vi "Image.vi"() -> ()   [LabVIEW 2017]
uses:
  ZaberTSeriesVI/Public/Utility/Request.ctl
  <vilib>/DAQmx/write.llb/DAQmx Write (Digital Bool 1Line 1Point).vi
  <vilib>/DAQmx/write.llb/DAQmx Write (Analog DBL 1Chan 1Samp).vi
  <vilib>/DAQmx/create/channels.llb/DAQmx Create Channel (AO-Voltage-Basic).vi
  <vilib>/DAQmx/miscellaneous.llb/DAQmx Fill In Error Info.vi
  <vilib>/DAQmx/create/channels.llb/DAQmx Create Channel (DO-Digital Output).vi
  <vilib>/Utility/file.llb/Read Delimited Spreadsheet (DBL).vi
  <vilib>/Utility/file.llb/Write Delimited Spreadsheet (string).vi
  <vilib>/Analysis/Matrix/Numeric/Conversions/Matrix To Array - RM.vi
  ZaberTSeriesVI/ZaberTSeries.lvlib
  <vilib>/Analysis/NI_AALPro.lvlib
  <vilib>/Analysis/Matrix/NI_Matrix.lvlib
panel:
  in  "Maximum offset":dbl=0.5
  out "WriteMS":bool=TRUE
  in  "Select PORT for LCQ":tag
  out "error out MS":errorcluster
  out "DAQmx Task MS":refnum<k21>
  in  "Stop MS":bool
  in  "scan range y [1E-7m]":dbl=282879.0 min=20.0 max=282879.0 step=2.0
  in  "scan range x [1E-7m]":dbl=282879.0 min=20.0 max=282879.0 step=2.0
  in  "File Export Path":path
  out "z(x) corrected":i32
  out "x corrected":i32
  out "zs":i32
  out "ys":i32
  out "xs":i32
  in  "Starting point":bool
  in  "Justage":bool
  out "error out Laserdiode":errorcluster
  in  "Request 11":T1={"Device Number"=0, "Command"=0, "Data"=0, "Response Count"=1} {"Command" items=["Echo"=55, "Home"=1, "Move Absolute"=20, "Move Relative"=21, "Move at Constant Speed"=22, "Renumber"=2, "Restore Settings"=36, "Stop"=23]}
  out "error out Stage":errorcluster
  in  "Refresh Button":bool
  out "ready.":bool
  out "Offset z(y) per µm":dbl
  out "Offset z(x) per µm":dbl
  out "z 3":i32
  out "z 2":i32
  out "z 1":i32
  in  "z [1E-7m]":i32=26400 min=0 max=282879 step=2
  in  "return to startpoint":bool
  out "x 3":i32
  out "y 3":i32
  out "x 2":i32
  out "y 2":i32
  in  "?":bool
  in  "?":bool
  out "Offset y per µm":dbl
  out "Offset x per µm":dbl
  in  "Calc Offset":bool
  in  "calibration":bool
  in  "Lens":enum16{"5x", "10x", "20x", "40x"}(ring)
  out "Read?":bool
  in  "Calib Path":path
  in  "Read Calibration file?":bool
  in  "intercept":dbl
  in  "slope":dbl
  in  "Shutter time (ms)":dbl=1.0 min=1.0 max=100000.0 step=1.0
  in  "y = step height [1E-7m]":dbl=2.0 min=2.0 max=282879.0 step=2.0
  in  "step scanning or continous (scan speed)":bool
  in  "Scan speed in µm/s":dbl=2.0 min=0.0 max=1000.0 step=2.0
  in  "End measurement":bool
  in  "x = step width [1E-7m]":dbl=2.0 min=2.0 max=282879.0 step=2.0
  in  "Begin measurement":bool
  out "error out shutter":errorcluster
  in  "Open/Close Shutter":bool
  in  "Select Channel for Shutter":tag
  out "y 1":i32
  out "x 1":i32
  in  "Turn on / off":bool
  in  "Set Zero":bool
  in  "Stop Laser":bool
  in  "stop Shutter":bool
  in  "Laserpower [W]":dbl(slide)=1e-08 min=0.0 max=1.0 step=0.1 scale=0.0..0.6
  in  "Select Channel for Laserdiode":tag
  out "position reached":bool
  in  "x [1E-7m]":i32 min=0 max=282879 step=2
  in  "Move":bool
  in  "y [1E-7m]":i32 min=0 max=282879 step=2
  in  "Stop Button":bool
  in  "Initialize Stage":bool
  in  "Select COM Port for Stage":refnum<visa-resource-name>
  out "DAQmx Task Shutter":refnum<k21>
  out "DAQmx Task Name Diode":refnum<k21>
  # "Imaging"
  # "Port 1, Line 0 = PFI0/P1.0"
  # "Set shutter to Xgate and Shutter enabled. Set Laserdiode controller to 0 mA and on. Make sure the stages manual knobs are in zero position. For calibration, a tab delimiter is used.\nNo plausibility check is performed on the calibration file!"
  # "!!TAKE CARE OF 5x vs 40x!!"
  # "CAREFUL! Init. will also reset z axis!!"
  # "Step height is a function of the temperature drift by desorption. In 10s@1300mA, ~1mm diameter is desorbed.\nPlease note: With scan speed, the outer limits are not perfectly timed. This is a numeric and electric issue and cannot be resolved"
  # "need to match\nmeas time in .seq\nfile"
  # "Please note it's 1E-7, not 1E-6!!"
  # "Before beginning the measurement, make sure you have set a shutter time, step height and width. Set your starting point and the calibration manually using this program and a camera. Save the position as it will be used for reset within the measurement!!!! \nCalibration: Set the offset positions properly. Take in mind that the stage moves towards positive values, therefore (0,0,0) must be lower than (0,y,0) and so on.\nClose the shutter, turn off Justage, then Turn on laser with the desired laser power, then hit begin measurement. If in measurement, the laser or shutter can be turned off using \"turn on/off\" button and the measurement can be stopped per axis using \"STOP\"."
  # "Offset listing"
  # "!!!! Set the calibration file for the laser power in backend: It is valid only for a specific optical path. Calibrate the laser power to the current in the experiment (have been measured for LD setup with microscope optics), then calculate intercept and slope and enter it as \"b\" and \"m\" according to y = mx+b in backend"
  # "0.5W = c.a. 900mA"
  # "This VI corrects the offset of the setup and substrate (e.g. rotation in the coating, tilt of slides,..) and the stage itself (1.2% moving too less per axis). The error in laser focus is additive in both x and y tilts and corrected as well. The stage error in z axis is only minor and cannot be corrected (1.2% of 100µm are 1.2µm < stage resolution - and this is already quite a lot)"
  # "x-, and y-value should be visible here, stating the current position (indicated by green light). \"Set zero\" sets the stage to absolute zero, but does not stop the measurement! \"Return to corrected zero\" returns the stage to bufff (x,y,z) = (0,0,0) starting point.  \"Calc offset\" corrects the xy- and xz-divergence on the spots and laser beam divergence on the substrate according to manually set calibration points.\n \nIf the measurements has finished, \"Begin measurement\" will go off and the stage will reset to buffered (x;y) or zero.\n\nSometimes the read current position will return the storing command. I don't know why. Workaround: Hit the button once more\n\nPlease note that if you pick scan speed, no export file will be written. From your starting point, the laser continously scans the substrate using the user-defined scan speed. The maximum travel distance of the stage is 28.2879 mm, minus the starting point, if defined. If required, remember that s=v*t.\n\nIf no export path is specified, the default path will be C:\\Users\\Username\\Documents\\LabVIEW Data\\"
  # "correct z with new justage"
  # "Bugtracker"
  # "Check laser spot correction in z with camera\n\nRead out current position sometimes returns\nreadout command\n."
  # "\"Maximum offset\" is the value that should not be exceed in the offset listing by any entry.\nAdjust only if necessary!"
  # "Zero corrected:"
  # "Disclaimer\nThis VI has not been excessively\ntested for safe use. Please use\nwith great care. \nalpha version without optimization"
  # "xz alignment:"
  # "yz alignment:"
  # "Error code stage:\n1 \tCannot Home \tHome - Device has traveled a long distance without triggering the home sensor. Device may be stalling or slipping.\n2 \tDevice Number Invalid \tRenumbering data out of range.\n14 \tVoltage Low \tPower supply voltage too low.\n15 \tVoltage High \tPower supply voltage too high.\n18 \tStored Position Invalid \tThe position stored in the requested register is no longer valid. This is probably because the maximum range was reduced.\n20 \tAbsolute Position Invalid \tMove Absolute - Target position out of range.\n21 \tRelative Position Invalid \tMove Relative - Target position out of range.\n22 \tVelocity Invalid \tConstant velocity move. Velocity out of range.\n36 \tPeripheral Id Invalid \tRestore Settings - peripheral id is invalid. Please use one of the peripheral ids listed in the user manual, or 0 for default.\n37 \tResolution Invalid \tInvalid microstep resolution. Resolution may only be 1, 2, 4, 8, 16, 32, 64, 128.\n38 \tRun Current Invalid \tRun current out of range. See command 38 for allowable values.\n39 \tHold Current Invalid \tHold current out of range. See command 39 for allowable values.\n40 \tMode Invalid \tSet Device Mode - one or more of the mode bits is invalid.\n41 \tHome Speed Invalid \tHome speed out of range. The range of home speed is determined by the resolution.\n42 \tSpeed Invalid \tTarget speed out of range. The range of target speed is determined by the resolution.\n43 \tAcceleration Invalid \tTarget acceleration out of range. The range of target acceleration is determined by the resolution.\n44 \tMaximum Range Invalid \tThe maximum range may only be set between 1 and the resolution limit of the stepper controller, which is 16,777,215.\n45 \tCurrent Position Invalid \tCurrent position out of range. Current position must be between 0 and the maximum range.\n46 \tMaximum Relative Move Invalid \tMax relative move out of range. Must be between 0 and 16,777,215.\n47 \tOffset Invalid \tHome offset out of range. Home offset must be between 0 and maximum range.\n48 \tAlias Invalid \tAlias out of range.\n49 \tLock State Invalid \tLock state must be 1 (locked) or 0 (unlocked).\n53 \tSetting Invalid \tReturn Setting - data entered is not a valid setting command number. Valid setting command numbers are the command numbers of any \"Set ...\" instructions.\n64 \tCommand Invalid \tCommand number not valid in this firmware version.\n255 \tBusy \tAnother command is executing and cannot be pre-empted. Either stop the previous command or wait until it finishes before trying again.\n1600 \tSave Position Invalid \tSave Current Position register out of range (must be 0-15).\n1601 \tSave Position Not Homed \tSave Current Position is not allowed unless the device has been homed.\n1700 \tReturn Position Invalid \tReturn Stored Position register out of range (must be 0-15).\n1800 \tMove Position Invalid \tMove to Stored Position register out of range (must be 0-15).\n1801 \tMove Position Not Homed \tMove to Stored Position is not allowed unless the device has been homed.\n2146 \tRelative Position Limited \tMove Relative (command 20) exceeded maximum relative move range. Either move a shorter distance, or change the maximum relative move (command 46).\n3600 \tSettings Locked \tMust clear Lock State (command 49) first. See the Set Lock State command for details.\n4008 \tDisable Auto Home Invalid \tSet Device Mode - this is a linear actuator; Disable Auto Home is used for rotary actuators only.\n4010 \tBit 10 Invalid \tSet Device Mode - bit 10 is reserved and must be 0.\n4012 \tHome Switch Invalid \tSet Device Mode - this device has integrated home sensor with preset polarity; mode bit 12 cannot be changed by the user.\n4013 \tBit 13 Invalid \tSet Device Mode - bit 13 is reserved and must be 0."
  # "Copyright (c) 2020 Alexander Knodel\n\nPermission is hereby granted, free of charge, to any person obtaining a copy\nof this software and associated documentation files (the \"Software\"), to deal\nin the Software without restriction, including without limitation the rights\nto use, copy, modify, merge, publish, distribute, sublicense, and/or sell\ncopies of the Software, and to permit persons to whom the Software is\nfurnished to do so, subject to the following conditions:\n\nThe above copyright notice and this permission notice shall be included in all\ncopies or substantial portions of the Software.\n\nTHE SOFTWARE IS PROVIDED \"AS IS\", WITHOUT WARRANTY OF ANY KIND, EXPRESS OR\nIMPLIED, INCLUDING BUT NOT LIMITED TO THE WARRANTIES OF MERCHANTABILITY,\nFITNESS FOR A PARTICULAR PURPOSE AND NONINFRINGEMENT. IN NO EVENT SHALL THE\nAUTHORS OR COPYRIGHT HOLDERS BE LIABLE FOR ANY CLAIM, DAMAGES OR OTHER\nLIABILITY, WHETHER IN AN ACTION OF CONTRACT, TORT OR OTHERWISE, ARISING FROM,\nOUT OF OR IN CONNECTION WITH THE SOFTWARE OR THE USE OR OTHER DEALINGS IN THE\nSOFTWARE."
types:
  T1 = typedef "ZaberTSeries.lvlib/Request.ctl" = cluster{"Device Number":u8, "Command":u8, "Data":i32, "Response Count":i32}
  T2 = typedef "ZaberTSeries.lvlib/Response.ctl" = cluster{"Device Number":u8, "Command":u8, "Data":i32}
  T3 = typedef "NI_Matrix.lvlib/RealMatrix.ctl" = dbl[][]
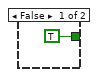
[diagram p2: hidden frame]
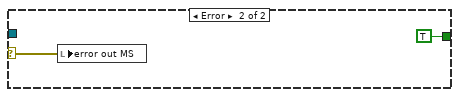
[diagram p3: hidden frame]
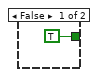
[diagram p4: hidden frame]
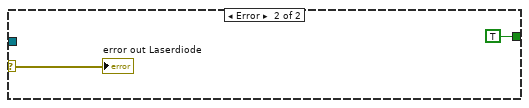
[diagram p5: hidden frame]
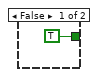
[diagram p6: hidden frame]
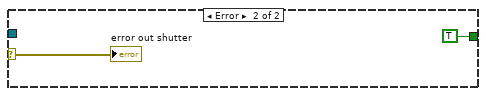
[diagram p7: hidden frame]
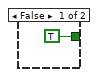
[diagram p8: hidden frame]
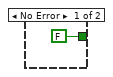
[diagram p9: hidden frame]
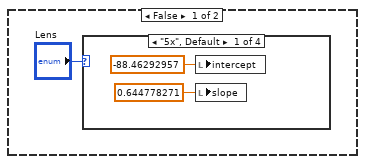
[diagram p10: hidden frame]
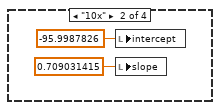
[diagram p11: hidden frame]
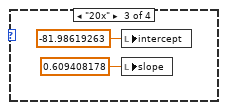
[diagram p12: hidden frame]
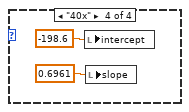
[diagram p13: hidden frame]
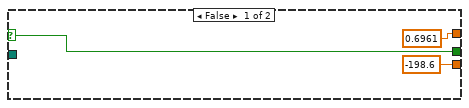
[diagram p14: hidden frame]
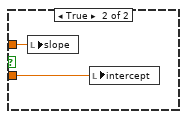
[diagram p15: hidden frame]
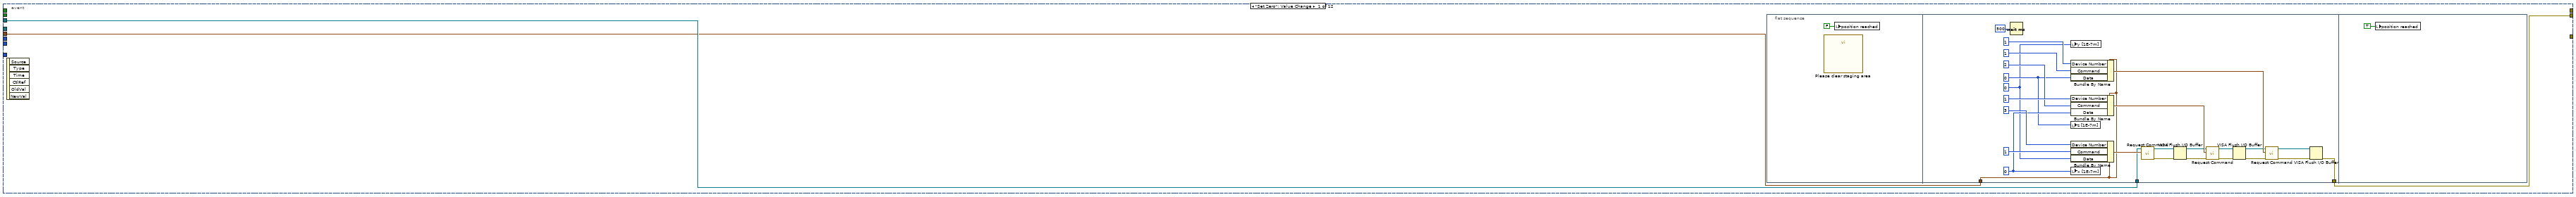
[diagram p16: hidden frame]
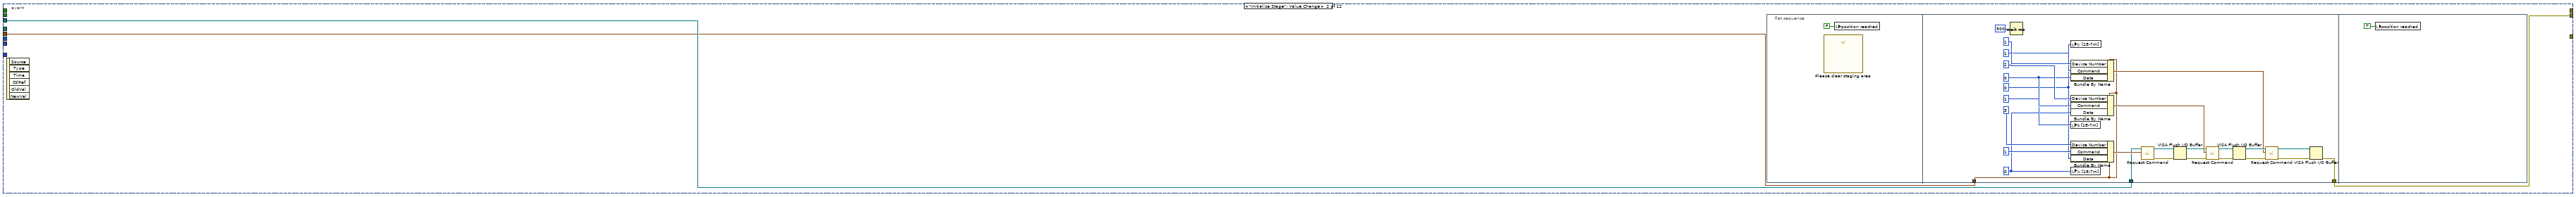
[diagram p17: hidden frame]
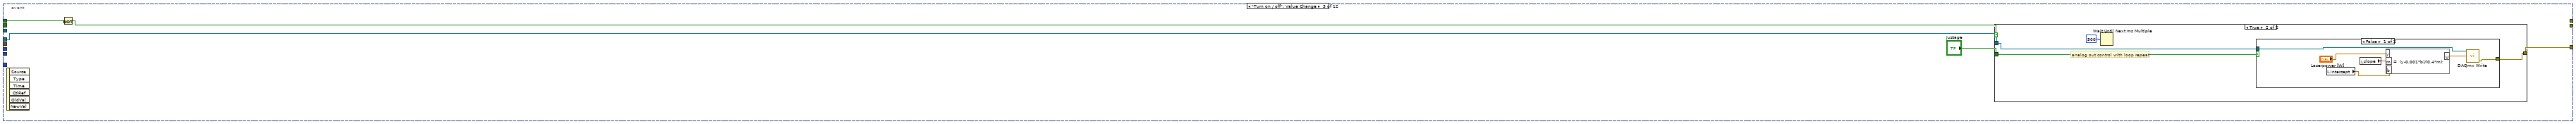
[diagram p18: hidden frame]
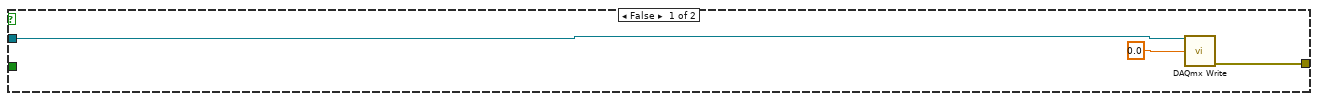
[diagram p19: hidden frame]
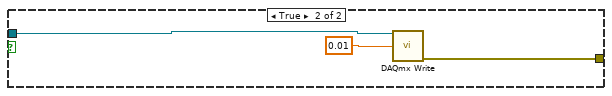
[diagram p20: hidden frame]
diagram:
  n1 = flat-sequence {
    tunnel: [w4] -> w2
    tunnel: w2 -> [w86]
    tunnel: [w86] -> w1
    tunnel: w1 -> [_]
    frame #0 {
      n2 = control-ref of="This VI"() -> (w3:refnum<vi>)
      n3 = invoke class="VI" method="Default Vals.Reinit All"(reference=w3) -> ()  [unwired: 2 in, 3 out]
    }
    frame #1 {
      n4 = while {
        stop <- w8 continue-if-true
        n5 = local read "Initialize Stage"() -> (w5:bool)
        n6 = Wait Until Next ms Multiple(millisecond multiple=u32 500) -> ()  [unwired: 1 out]
        n7 = case shown="True" w5 {
          tunnel: [TRUE w14] -> w7
          tunnel: "Select PORT for LCQ" -> [_ w13]
          frame False {
          }
          frame True {
            n8 = call-poly <vilib>:"DAQmx Create Virtual Channel.vi"("lines"=w13) -> ("task out"=w17:refnum<k21>, "error out"=w18:errorcluster)  [unwired: 13 in]
            n9 = call <vilib>:"DAQmx Start Task.vi"("task/channels in"=w17, "error in"=w18) -> ("task out"=w15:refnum<k21>, "error out"=w16:errorcluster)  [unwired: 12 in]
            "DAQmx Task MS" <- w15
            n10 = case shown="No Error" w16 {
              selector: w16 -> [_ w25]
              tunnel: w15 -> [w22 _]
              tunnel: [FALSE TRUE] -> w14
              frame No Error {
                n11 = call-poly <vilib>:"DAQmx Write.vi"("task/channels in"=w22, "data"=FALSE) -> ("error out"=→"error out MS":errorcluster)  [unwired: 11 in, 2 out]
                "WriteMS" <- TRUE
              }
              frame Error {
                n12 = local write "error out MS"(w25) -> ()
              }
            }
          }
        }
        n13 = Not(x="Stop MS") -> (.not. x?=w9:bool)
        n14 = And(x=w7, y=w9) -> (x .and. y?=w8:bool)
      }
      n15 = while {
        stop <- w27 continue-if-true
        # "initializes Slide Control to 0"
        n16 = Wait Until Next ms Multiple(millisecond multiple=u32 500) -> ()  [unwired: 1 out]
        n17 = local read "Initialize Stage"() -> (w26:bool)
        n18 = case shown="True" w26 {
          tunnel: "Select Channel for Laserdiode" -> [_ w37]
          tunnel: [TRUE w35] -> w31
          frame False {
          }
          frame True {
            n19 = call-poly <vilib>:"DAQmx Create Virtual Channel.vi"("physical channels"=w37) -> ("task out"=w39:refnum<k21>, "error out"=w38:errorcluster)  [unwired: 13 in]
            n20 = call <vilib>:"DAQmx Start Task.vi"("task/channels in"=w39, "error in"=w38) -> ("task out"=w34:refnum<k21>, "error out"=w36:errorcluster)  [unwired: 12 in]
            "DAQmx Task Name Diode" <- w34
            n21 = case shown="No Error" w36 {
              selector: w36 -> [_ w44]
              tunnel: [FALSE TRUE] -> w35
              tunnel: w34 -> [w41 _]
              frame No Error {
                n22 = call-poly <vilib>:"DAQmx Write.vi"("task/channels in"=w41, "data"=0.0) -> ("error out"=w42:errorcluster)  [unwired: 11 in, 2 out]
                n23 = local write "error out Laserdiode"(w42) -> ()
              }
              frame Error {
                "error out Laserdiode" <- w44
              }
            }
          }
        }
        n24 = Not(x="Stop Laser") -> (.not. x?=w30:bool)
        n25 = And(x=w31, y=w30) -> (x .and. y?=w27:bool)
      }
      n26 = while {
        stop <- w50 continue-if-true
        # "initializes Slide Control to 0"
        n27 = Wait Until Next ms Multiple(millisecond multiple=u32 500) -> ()  [unwired: 1 out]
        n28 = local read "Initialize Stage"() -> (w46:bool)
        n29 = case shown="True" w46 {
          tunnel: "Select Channel for Shutter" -> [_ w56]
          tunnel: [TRUE w61] -> w49
          frame False {
          }
          frame True {
            # "Make sure Shutter in on, on X Gate and enabled"
            n30 = call-poly <vilib>:"DAQmx Create Virtual Channel.vi"("maximum value"=5.0, "minimum value"=0.0, "physical channels"=w56) -> ("task out"=w58:refnum<k21>, "error out"=w57:errorcluster)  [unwired: 11 in]
            n31 = call <vilib>:"DAQmx Start Task.vi"("task/channels in"=w58, "error in"=w57) -> ("task out"=w54:refnum<k21>, "error out"=w55:errorcluster)  [unwired: 12 in]
            "DAQmx Task Shutter" <- w54
            n32 = case shown="No Error" w55 {
              selector: w55 -> [_ w66]
              tunnel: [FALSE TRUE] -> w61
              tunnel: w54 -> [w64 _]
              frame No Error {
                n33 = call-poly <vilib>:"DAQmx Write.vi"("task/channels in"=w64, "data"=0.0) -> ("error out"=w63:errorcluster)  [unwired: 11 in, 2 out]
                n34 = local write "error out shutter"(w63) -> ()
              }
              frame Error {
                "error out shutter" <- w66
              }
            }
          }
        }
        n35 = Not(x="stop Shutter") -> (.not. x?=w51:bool)
        n36 = And(x=w49, y=w51) -> (x .and. y?=w50:bool)
      }
      n37 = while {
        tunnel: ["Stop Button"] -> w4
        stop <- w70 continue-if-true
        n38 = Wait Until Next ms Multiple(millisecond multiple=u32 500) -> ()  [unwired: 1 out]
        n39 = case shown="True" "Initialize Stage" {
          tunnel: [TRUE w82] -> w72
          tunnel: "Select COM Port for Stage" -> [_ w79]
          frame False {
          }
          frame True {
            n40 = call "Initialize.vi"("VISA resource name"=w79) -> ("error out"=w81:errorcluster, "VISA resource name out"=w76:refnum<visa-resource-name>)  [unwired: 8 in, 1 out]
            n41 = property class="Instr"(reference=w76, error in=w81, "Timeout"=u32 30000 ("General Settings:Timeout Value")) -> (reference out=w77:refnum<visa-resource-name>, error out=w78:errorcluster)
            n42 = local write "Select COM Port for Stage"(w77) -> ()
            n43 = case shown="Error" w78 {
              selector: w78 -> [_ w84]
              tunnel: [FALSE TRUE] -> w82
              frame No Error {
              }
              frame Error {
                "error out Stage" <- w84
              }
            }
          }
        }
        n44 = Not(x="Stop Button") -> (.not. x?=w71:bool)
        n45 = And(x=w72, y=w71) -> (x .and. y?=w70:bool)
      }
    }
    frame #2 {
      n46 = flat-sequence {
        frame #0 {
          n47 = case shown="True" "Read Calibration file?" {
            tunnel: "Calib Path" -> [_ w98]
            frame False {
              n48 = case shown="\"5x\", Default" "Lens" {
                frame "5x", Default {
                  n49 = local write "intercept"(-88.46292957 ("input variable")) -> ()
                  n50 = local write "slope"(0.644778271 ("input variable")) -> ()
                }
                frame "10x" {
                  n51 = local write "intercept"(-95.9987826 ("input variable")) -> ()
                  n52 = local write "slope"(0.709031415 ("input variable")) -> ()
                }
                frame "20x" {
                  n53 = local write "intercept"(-81.98619263 ("input variable")) -> ()
                  n54 = local write "slope"(0.609408178 ("input variable")) -> ()
                }
                frame "40x" {
                  n55 = local write "intercept"(-198.6 ("intercept")) -> ()
                  n56 = local write "slope"(0.6961 ("slope")) -> ()
                }
              }
            }
            frame True {
              n57 = flat-sequence {
                tunnel: [w103] -> w99
                tunnel: w98 -> [w103]
                tunnel: [w104] -> w102
                tunnel: [w108] -> w101
                tunnel: [w107] -> w100
                tunnel: w99 -> [w105]
                tunnel: w102 -> [w127]
                tunnel: w101 -> [w126]
                tunnel: w100 -> [w125]
                frame #0 {
                }
                frame #1 {
                  n58 = call <vilib>:"Is Path and Not Empty.vi"("path"=w105) -> ("Is Path and Not Empty?"=w109:bool)  [unwired: 4 in]
                  n59 = Wait (ms)(milliseconds to wait=u32 500) -> ()  [unwired: 1 out]
                  n60 = case shown="True" w109 {
                    selector: w109 -> [w110 _]
                    tunnel: w105 -> [_ w117]
                    tunnel: [0.6961 ("slope") w115] -> w107
                    tunnel: [-198.6 ("intercept") w116] -> w108
                    tunnel: [w110 w113] -> w104
                    frame False {
                    }
                    frame True {
                      n61 = call-poly <vilib>:"Read Delimited Spreadsheet.vi"("file path (dialog if empty)"=w117) -> ("all rows"=w120:dbl[][], "EOF?"=→"Read?":bool, "error out"=w118:errorcluster)  [unwired: 9 in, 3 out]
                      n62 = local write "error out Laserdiode"(w118) -> ()
                      n63 = Index Array(array=w120, index (col)=1 ("disabled index (col)")) -> (element=w124:dbl[])  [unwired: 1 in]
                      n64 = Index Array(array=w120, index (col)=0 ("disabled index (col)")) -> (element=w123:dbl[])  [unwired: 1 in]
                      n65 = call <vilib>:"Linear Fit.vi"("Y"=w124, "X"=w123) -> ("slope"=w115:dbl, "intercept"=w116:dbl)  [unwired: 9 in, 3 out]
                      n66 = Not A Number/Path/Refnum?(number/path/refnum=w116) -> (NaN/Path/Refnum?=w114:bool)
                      n67 = Not(x=w114) -> (.not. x?=w113:bool)
                    }
                  }
                }
                frame #2 {
                  n68 = case shown="False" w127 {
                    tunnel: w126 -> [_ w130]
                    tunnel: w125 -> [_ w131]
                    frame False {
                      n69 = call "Display Message to User"() -> ()  [unwired: 10 in, 2 out]
                      n70 = local write "intercept"(-198.6 ("intercept")) -> ()
                      n71 = local write "slope"(0.6961 ("slope")) -> ()
                    }
                    frame True {
                      n72 = local write "slope"(w131) -> ()
                      n73 = local write "intercept"(w130) -> ()
                    }
                  }
                }
              }
            }
          }
        }
      }
    }
    frame #3 {
      n74 = flat-sequence {
        tunnel: [w137] -> w133
        tunnel: [w134] -> w132
        tunnel: w133 -> [w1147]
        tunnel: w132 -> [w1146]
        frame #0 {
          n75 = local read "Select COM Port for Stage"() -> (w135:refnum<visa-resource-name>)
          n76 = while {
            tunnel: "Request 11" -> [w146]
            tunnel: w135 -> [w145]
            stop <- w147 stop-if-true
            n77 = local read "position reached"() -> (→"ready.":bool)
            n78 = local read "DAQmx Task Name Diode"() -> (w139:refnum<k21>)
            n79 = Wait Until Next ms Multiple(millisecond multiple=u32 500) -> ()  [unwired: 1 out]
            n80 = Not(x="Open/Close Shutter") -> (.not. x?=w142:bool)
            n81 = event shown="[9] \"Refresh Button\": Value Change" {
              selector: _ -> [_ _ _ _ _ _ _ _ _ _ _ _]
              dyn-events: _ -> [_ _ _ _ _ _ _ _ _ _ _ _]
              timeout: _ -> [_ _ _ _ _ _ _ _ _ _ _ _]
              tunnel: [w154 w185 _ w237 _ _ _ _ w322 w353 _ w447] -> w144
              tunnel: w145 -> [w155 w186 _ w238 _ _ _ _ w321 w352 _ w448]
              tunnel: "x [1E-7m]" -> [_ _ _ _ w307 w309 w312 w315 w320 _ _ _]
              tunnel: "y [1E-7m]" -> [_ _ _ _ w306 w310 w313 w316 w319 _ _ _]
              tunnel: "z [1E-7m]" -> [_ _ _ _ w305 w308 w311 w314 w318 _ _ _]
              tunnel: w142 -> [_ _ _ _ _ _ _ _ _ _ w443 _]
              tunnel: w146 -> [w153 w184 _ w236 _ _ _ _ w317 w351 _ w446]
              tunnel: [_ _ _ _ _ _ _ _ _ _ w440 _] -> w141
              tunnel: "Turn on / off" -> [_ _ w217 _ _ _ _ _ _ _ _ _]
              tunnel: [_ _ w219 _ _ _ _ _ _ _ _ _] -> w140
              tunnel: w139 -> [_ _ w218 _ _ _ _ _ _ _ _ _]
              event "Set Zero": Value Change {
                n82 = event-data() -> ()  [unwired: 1 in, 6 out]
                n83 = flat-sequence {
                  tunnel: w155 -> [w166]
                  tunnel: [w163] -> w154
                  tunnel: w153 -> [w160]
                  frame #0 {
                    n84 = call "Please clear staging area"() -> ()  [unwired: 18 in, 2 out]
                    n85 = local write "position reached"(FALSE ("Blinking")) -> ()
                  }
                  frame #1 {
                    w158 = 0 ("y-value 2")
                    w159 = 0 ("y-value 2")
                    w157 = 0 ("x-value 2")
                    n86 = Wait (ms)(milliseconds to wait=u32 500 ("millisecond timer value")) -> ()  [unwired: 1 out]
                    n87 = local write "y [1E-7m]"(w157) -> ()
                    n88 = Bundle By Name(cluster=w160, "Device Number"=u8 1, "Command"=u8 1, "Data"=w158) -> (w168:T1)
                    n89 = Bundle By Name(cluster=w160, "Device Number"=u8 2, "Command"=u8 1, "Data"=w159) -> (w177:T1)
                    n90 = local write "z [1E-7m]"(w158) -> ()
                    n91 = Bundle By Name(cluster=w160, "Device Number"=u8 3, "Command"=u8 1, "Data"=w157) -> (w180:T1)
                    n92 = local write "x [1E-7m]"(w159) -> ()
                    n93 = call "Request Command.vi"("Request"=w180, "VISA resource name"=w166) -> ("error out"=w182:errorcluster, "VISA resource name out"=w181:refnum<visa-resource-name>)  [unwired: 6 in, 2 out]
                    n94 = VISA Flush I/O Buffer(VISA resource name=w181, error in (no error)=w182) -> (VISA resource name out=w176:refnum<visa-resource-name>, error out=w175:errorcluster)  [unwired: 1 in]
                    n95 = call "Request Command.vi"("error in (no error)"=w175, "Request"=w177, "VISA resource name"=w176) -> ("error out"=w171:errorcluster, "VISA resource name out"=w172:refnum<visa-resource-name>)  [unwired: 5 in, 2 out]
                    n96 = VISA Flush I/O Buffer(VISA resource name=w172, error in (no error)=w171) -> (VISA resource name out=w164:refnum<visa-resource-name>, error out=w162:errorcluster)  [unwired: 1 in]
                    n97 = call "Request Command.vi"("error in (no error)"=w162, "Request"=w168, "VISA resource name"=w164) -> ("error out"=w165:errorcluster, "VISA resource name out"=w167:refnum<visa-resource-name>)  [unwired: 5 in, 2 out]
                    n98 = VISA Flush I/O Buffer(VISA resource name=w167, error in (no error)=w165) -> (error out=w163:errorcluster)  [unwired: 1 in, 1 out]
                  }
                  frame #2 {
                    n99 = local write "position reached"(TRUE ("Blinking")) -> ()
                  }
                }
              }
              event "Initialize Stage": Value Change {
                n100 = event-data() -> ()  [unwired: 1 in, 6 out]
                n101 = flat-sequence {
                  tunnel: w186 -> [w201]
                  tunnel: [w198] -> w185
                  tunnel: w184 -> [w191]
                  frame #0 {
                    n102 = call "Please clear staging area"() -> ()  [unwired: 18 in, 2 out]
                    n103 = local write "position reached"(FALSE ("Blinking")) -> ()
                  }
                  frame #1 {
                    w190 = 0 ("Data")
                    w189 = 0 ("y-value 2")
                    w188 = 0 ("x-value 2")
                    n104 = Wait (ms)(milliseconds to wait=u32 500 ("millisecond timer value")) -> ()  [unwired: 1 out]
                    n105 = local write "y [1E-7m]"(w188) -> ()
                    n106 = Bundle By Name(cluster=w191, "Device Number"=u8 1, "Command"=u8 1, "Data"=w190) -> (w193:T1)
                    n107 = Bundle By Name(cluster=w191, "Device Number"=u8 2, "Command"=u8 1, "Data"=w189) -> (w208:T1)
                    n108 = local write "z [1E-7m]"(w190) -> ()
                    n109 = Bundle By Name(cluster=w191, "Device Number"=u8 3, "Command"=u8 1, "Data"=w188) -> (w211:T1)
                    n110 = local write "x [1E-7m]"(w189) -> ()
                    n111 = call "Request Command.vi"("Request"=w211, "VISA resource name"=w201) -> ("error out"=w213:errorcluster, "VISA resource name out"=w212:refnum<visa-resource-name>)  [unwired: 6 in, 2 out]
                    n112 = VISA Flush I/O Buffer(VISA resource name=w212, error in (no error)=w213) -> (VISA resource name out=w207:refnum<visa-resource-name>, error out=w206:errorcluster)  [unwired: 1 in]
                    n113 = call "Request Command.vi"("error in (no error)"=w206, "Request"=w208, "VISA resource name"=w207) -> ("error out"=w202:errorcluster, "VISA resource name out"=w203:refnum<visa-resource-name>)  [unwired: 5 in, 2 out]
                    n114 = VISA Flush I/O Buffer(VISA resource name=w203, error in (no error)=w202) -> (VISA resource name out=w194:refnum<visa-resource-name>, error out=w195:errorcluster)  [unwired: 1 in]
                    n115 = call "Request Command.vi"("error in (no error)"=w195, "Request"=w193, "VISA resource name"=w194) -> ("error out"=w196:errorcluster, "VISA resource name out"=w197:refnum<visa-resource-name>)  [unwired: 5 in, 2 out]
                    n116 = VISA Flush I/O Buffer(VISA resource name=w197, error in (no error)=w196) -> (error out=w198:errorcluster)  [unwired: 1 in, 1 out]
                  }
                  frame #2 {
                    n117 = local write "position reached"(TRUE ("Blinking")) -> ()
                  }
                }
              }
              event "Turn on / off": Value Change {
                n118 = event-data() -> ()  [unwired: 1 in, 6 out]
                n119 = Not(x=w217) -> (.not. x?=w216:bool)
                n120 = case shown="True" w216 {
                  tunnel: w218 -> [w222 w225]
                  tunnel: [w220 w224] -> w219
                  tunnel: "Justage" -> [_ w223]
                  frame False {
                    n121 = call-poly <vilib>:"DAQmx Write.vi"("task/channels in"=w222, "data"=0.0) -> ("error out"=w220:errorcluster)  [unwired: 11 in, 2 out]
                  }
                  frame True {
                    # "analog out control with loop repeat"
                    n122 = Wait Until Next ms Multiple(millisecond multiple=u32 500) -> ()  [unwired: 1 out]
                    n123 = case shown="False" w223 {
                      tunnel: [w229 w234] -> w224
                      tunnel: w225 -> [w227 w235]
                      frame False {
                        n124 = local read "intercept"() -> (w230:dbl)
                        n125 = local read "slope"() -> (w231:dbl)
                        n126 = formula code="U =  (y-0.001*b)/(0.4*m);"("y"="Laserpower [W]", "m"=w231, "b"=w230) -> ("U"=w228:dbl)
                        n127 = call-poly <vilib>:"DAQmx Write.vi"("task/channels in"=w227, "data"=w228) -> ("error out"=w229:errorcluster)  [unwired: 11 in, 2 out]
                      }
                      frame True {
                        n128 = call-poly <vilib>:"DAQmx Write.vi"("task/channels in"=w235, "data"=0.01) -> ("error out"=w234:errorcluster)  [unwired: 11 in, 2 out]
                      }
                    }
                  }
                }
              }
              event "return to startpoint": Value Change {
                n129 = event-data() -> ()  [unwired: 1 in, 6 out]
                n130 = flat-sequence {
                  tunnel: w238 -> [w257]
                  tunnel: [w254] -> w237
                  tunnel: w236 -> [w251]
                  frame #0 {
                    n131 = local write "position reached"(FALSE ("Blinking")) -> ()
                  }
                  frame #1 {
                    n132 = local read "zs"() -> (w244:i32)
                    n133 = local read "xs"() -> (w245:i32)
                    n134 = local read "ys"() -> (w243:i32)
                    n135 = Wait (ms)(milliseconds to wait=u32 500 ("millisecond timer value")) -> ()  [unwired: 1 out]
                    n136 = Not Equal To 0?(x=w244) -> (x != 0?=w248:bool)
                    n137 = Not Equal To 0?(x=w245) -> (x != 0?=w250:bool)
                    n138 = Not Equal To 0?(x=w243) -> (x != 0?=w249:bool)
                    n139 = Build Array(w250, w249, w248) -> (w247:bool[])
                    n140 = And Array Elements(Boolean array=w247) -> (logical AND=w246:bool)
                    n141 = case shown="True" w246 {
                      tunnel: [w275 w301] -> w241
                      tunnel: [w274 w302] -> w240
                      tunnel: [w278 w303] -> w242
                      tunnel: w245 -> [_ w303]
                      tunnel: w243 -> [_ w302]
                      tunnel: w244 -> [_ w301]
                      frame False {
                        n142 = local read "z 1"() -> (w276:i32)
                        n143 = local read "x 1"() -> (w279:i32)
                        n144 = local read "y 1"() -> (w277:i32)
                        n145 = Build Array(w279, w277, w276) -> (w282:i32[])
                        n146 = Not Equal To 0?(x=w282) -> (x != 0?=w281:bool[])
                        n147 = And Array Elements(Boolean array=w281) -> (logical AND=w280:bool)
                        n148 = case shown="True" w280 {
                          tunnel: [w288 w300] -> w278
                          tunnel: w279 -> [_ w300]
                          tunnel: w277 -> [_ w299]
                          tunnel: [w286 w299] -> w274
                          tunnel: w276 -> [_ w298]
                          tunnel: [w284 w298] -> w275
                          frame False {
                            n149 = local read "error out Stage"() -> (w291:errorcluster)
                            n150 = call "Warning! You may ruin your measurement (no start. point)"("error in (no error)"=w291) -> ("z"=w285:dbl, "y"=w287:dbl, "x"=w289:dbl, "OK"=w283:bool, "error out"=w290:errorcluster)  [unwired: 14 in]
                            n151 = local write "error out Stage"(w290) -> ()
                            n152 = case shown="True" w283 {
                              tunnel: w289 -> [_ w295]
                              tunnel: [w292 w295] -> w288
                              tunnel: [w292 w294] -> w286
                              tunnel: w287 -> [_ w294]
                              tunnel: w285 -> [_ w293]
                              tunnel: [w292 w293] -> w284
                              frame False {
                                w292 = 0
                              }
                              frame True {
                              }
                            }
                          }
                          frame True {
                            n153 = local read "error out Stage"() -> (w297:errorcluster)
                            n154 = call "Display Message to User4"("error in (no error)"=w297) -> ("error out"=w296:errorcluster)  [unwired: 9 in, 1 out]
                            n155 = local write "error out Stage"(w296) -> ()
                          }
                        }
                      }
                      frame True {
                      }
                    }
                    n156 = local write "z [1E-7m]"(w241) -> ()
                    n157 = local write "x [1E-7m]"(w242) -> ()
                    n158 = local write "y [1E-7m]"(w240) -> ()
                    n159 = Bundle By Name(cluster=w251, "Device Number"=u8 1, "Command"=u8 20, "Data"=w241) -> (w259:T1)
                    n160 = Bundle By Name(cluster=w251, "Device Number"=u8 2, "Command"=u8 20, "Data"=w242) -> (w268:T1)
                    n161 = Bundle By Name(cluster=w251, "Device Number"=u8 3, "Command"=u8 20, "Data"=w240) -> (w271:T1)
                    n162 = call "Request Command.vi"("Request"=w271, "VISA resource name"=w257) -> ("error out"=w273:errorcluster, "VISA resource name out"=w272:refnum<visa-resource-name>)  [unwired: 6 in, 2 out]
                    n163 = VISA Flush I/O Buffer(VISA resource name=w272, error in (no error)=w273) -> (VISA resource name out=w267:refnum<visa-resource-name>, error out=w266:errorcluster)  [unwired: 1 in]
                    n164 = call "Request Command.vi"("error in (no error)"=w266, "Request"=w268, "VISA resource name"=w267) -> ("error out"=w262:errorcluster, "VISA resource name out"=w263:refnum<visa-resource-name>)  [unwired: 5 in, 2 out]
                    n165 = VISA Flush I/O Buffer(VISA resource name=w263, error in (no error)=w262) -> (VISA resource name out=w255:refnum<visa-resource-name>, error out=w253:errorcluster)  [unwired: 1 in]
                    n166 = call "Request Command.vi"("error in (no error)"=w253, "Request"=w259, "VISA resource name"=w255) -> ("error out"=w256:errorcluster, "VISA resource name out"=w258:refnum<visa-resource-name>)  [unwired: 5 in, 2 out]
                    n167 = VISA Flush I/O Buffer(VISA resource name=w258, error in (no error)=w256) -> (error out=w254:errorcluster)  [unwired: 1 in, 1 out]
                  }
                  frame #2 {
                    n168 = local write "position reached"(TRUE ("Blinking")) -> ()
                  }
                }
              }
              event "calibration": Value Change {
                n169 = event-data() -> ()  [unwired: 1 in, 6 out]
                "x 1" <- w307
                "y 1" <- w306
                "z 1" <- w305
              }
              event Value Change {
                n170 = event-data() -> ()  [unwired: 1 in, 6 out]
                "y 2" <- w310
                "x 2" <- w309
                "z 2" <- w308
              }
              event Value Change {
                n171 = event-data() -> ()  [unwired: 1 in, 6 out]
                "x 3" <- w312
                "y 3" <- w313
                "z 3" <- w311
              }
              event "Starting point": Value Change {
                n172 = event-data() -> ()  [unwired: 1 in, 6 out]
                "zs" <- w314
                "ys" <- w316
                "xs" <- w315
              }
              event "Move": Value Change {
                n173 = event-data() -> ()  [unwired: 1 in, 5 out]
                n174 = flat-sequence {
                  tunnel: [w336] -> w322
                  tunnel: w321 -> [w337]
                  tunnel: w320 -> [w324]
                  tunnel: w319 -> [w325]
                  tunnel: w318 -> [w326]
                  tunnel: w317 -> [w327]
                  frame #0 {
                    n175 = local write "position reached"(FALSE ("Blinking")) -> ()
                  }
                  frame #1 {
                    n176 = Wait (ms)(milliseconds to wait=u32 500 ("millisecond timer value")) -> ()  [unwired: 1 out]
                    n177 = Bundle By Name(cluster=w327, "Device Number"=u8 1, "Command"=u8 20, "Data"=w326) -> (w331:T1)
                    n178 = Bundle By Name(cluster=w327, "Device Number"=u8 2, "Command"=u8 20, "Data"=w324) -> (w344:T1)
                    n179 = Bundle By Name(cluster=w327, "Device Number"=u8 3, "Command"=u8 20, "Data"=w325) -> (w347:T1)
                    n180 = call "Request Command.vi"("Request"=w347, "VISA resource name"=w337) -> ("error out"=w349:errorcluster, "VISA resource name out"=w348:refnum<visa-resource-name>)  [unwired: 6 in, 2 out]
                    n181 = VISA Flush I/O Buffer(VISA resource name=w348, error in (no error)=w349) -> (VISA resource name out=w343:refnum<visa-resource-name>, error out=w342:errorcluster)  [unwired: 1 in]
                    n182 = call "Request Command.vi"("error in (no error)"=w342, "Request"=w344, "VISA resource name"=w343) -> ("error out"=w338:errorcluster, "VISA resource name out"=w339:refnum<visa-resource-name>)  [unwired: 5 in, 2 out]
                    n183 = VISA Flush I/O Buffer(VISA resource name=w339, error in (no error)=w338) -> (VISA resource name out=w333:refnum<visa-resource-name>, error out=w335:errorcluster)  [unwired: 1 in]
                    n184 = call "Request Command.vi"("error in (no error)"=w335, "Request"=w331, "VISA resource name"=w333) -> ("error out"=w334:errorcluster, "VISA resource name out"=w332:refnum<visa-resource-name>)  [unwired: 5 in, 2 out]
                    n185 = VISA Flush I/O Buffer(VISA resource name=w332, error in (no error)=w334) -> (error out=w336:errorcluster)  [unwired: 1 in, 1 out]
                  }
                  frame #2 {
                    n186 = local write "position reached"(TRUE ("Blinking")) -> ()
                  }
                }
              }
              event "Refresh Button": Value Change {
                n187 = event-data() -> ()  [unwired: 1 in, 6 out]
                n188 = while {
                  tunnel: [w360] -> w353
                  tunnel: w352 -> [w359]
                  tunnel: w351 -> [w358]
                  i -> [w356]
                  stop <- w354 continue-if-true
                  n189 = Equal?(x=w356, y=4.0) -> (x = y?=w355:bool)
                  n190 = flat-sequence {
                    tunnel: [w366] -> w360
                    tunnel: w355 -> [w362]
                    tunnel: w359 -> [w365]
                    tunnel: w358 -> [w364]
                    tunnel: [w361] -> w354
                    frame #0 {
                      n191 = flat-sequence {
                        tunnel: [w372] -> w368
                        tunnel: [w371] -> w367
                        tunnel: w365 -> [w370]
                        tunnel: w364 -> [w369]
                        tunnel: w368 -> [w398]
                        tunnel: w367 -> [w397]
                        tunnel: w364 -> [w396]
                        tunnel: [w399] -> w363
                        tunnel: [w438] -> w366
                        tunnel: w363 -> [w438]
                        tunnel: w362 -> [w437]
                        tunnel: [w430] -> w361
                        frame #0 {
                          n192 = Bundle By Name(cluster=w369, "Device Number"=u8 3, "Command"=u8 16, "Data"=2) -> (w393:T1)
                          n193 = Bundle By Name(cluster=w369, "Device Number"=u8 2, "Command"=u8 16, "Data"=1) -> (w387:T1)
                          n194 = Bundle By Name(cluster=w369, "Device Number"=u8 1, "Command"=u8 16, "Data"=0) -> (w383:T1)
                          n195 = Wait (ms)(milliseconds to wait=u32 2000 ("millisecond timer value")) -> ()  [unwired: 1 out]
                          n196 = call "Request Command.vi"("Request"=w383, "VISA resource name"=w370) -> ("error out"=w381:errorcluster, "VISA resource name out"=w382:refnum<visa-resource-name>)  [unwired: 6 in, 2 out]
                          n197 = VISA Flush I/O Buffer(VISA resource name=w382, error in (no error)=w381) -> (VISA resource name out=w376:refnum<visa-resource-name>, error out=w373:errorcluster)  [unwired: 1 in]
                          n198 = call "Request Command.vi"("error in (no error)"=w373, "Request"=w387, "VISA resource name"=w376) -> ("error out"=w388:errorcluster, "VISA resource name out"=w389:refnum<visa-resource-name>)  [unwired: 5 in, 2 out]
                          n199 = VISA Flush I/O Buffer(VISA resource name=w389, error in (no error)=w388) -> (VISA resource name out=w375:refnum<visa-resource-name>, error out=w374:errorcluster)  [unwired: 1 in]
                          n200 = call "Request Command.vi"("error in (no error)"=w374, "Request"=w393, "VISA resource name"=w375) -> ("error out"=w395:errorcluster, "VISA resource name out"=w394:refnum<visa-resource-name>)  [unwired: 5 in, 2 out]
                          n201 = VISA Flush I/O Buffer(VISA resource name=w394, error in (no error)=w395) -> (VISA resource name out=w371:refnum<visa-resource-name>, error out=w372:errorcluster)  [unwired: 1 in]
                        }
                        frame #1 {
                          n202 = Wait (ms)(milliseconds to wait=u32 2000 ("millisecond timer value")) -> ()  [unwired: 1 out]
                          n203 = Bundle By Name(cluster=w396, "Device Number"=u8 2, "Command"=u8 17, "Data"=1) -> (w409:T1)
                          n204 = Bundle By Name(cluster=w396, "Device Number"=u8 3, "Command"=u8 17, "Data"=2) -> (w424:T1)
                          n205 = Bundle By Name(cluster=w396, "Device Number"=u8 1, "Command"=u8 17, "Data"=0) -> (w423:T1)
                          n206 = call "Request Command.vi"("error in (no error)"=w398, "Request"=w423, "VISA resource name"=w397) -> ("error out"=w425:errorcluster, "First Response"=w412:T2, "VISA resource name out"=w428:refnum<visa-resource-name>)  [unwired: 5 in, 1 out]
                          n207 = Unbundle(w412) -> ("Data"=w410:i32)  [unwired: 2 out]
                          n208 = VISA Flush I/O Buffer(VISA resource name=w428, error in (no error)=w425) -> (VISA resource name out=w405:refnum<visa-resource-name>, error out=w404:errorcluster)  [unwired: 1 in]
                          n209 = local write "z [1E-7m]"(w410) -> ()
                          n210 = call "Request Command.vi"("error in (no error)"=w404, "Request"=w424, "VISA resource name"=w405) -> ("error out"=w426:errorcluster, "First Response"=w411:T2, "VISA resource name out"=w427:refnum<visa-resource-name>)  [unwired: 5 in, 1 out]
                          n211 = Unbundle(w411) -> ("Data"=w400:i32)  [unwired: 2 out]
                          n212 = VISA Flush I/O Buffer(VISA resource name=w427, error in (no error)=w426) -> (VISA resource name out=w402:refnum<visa-resource-name>, error out=w403:errorcluster)  [unwired: 1 in]
                          n213 = local write "y [1E-7m]"(w400) -> ()
                          n214 = call "Request Command.vi"("error in (no error)"=w403, "Request"=w409, "VISA resource name"=w402) -> ("error out"=w406:errorcluster, "First Response"=w407:T2, "VISA resource name out"=w408:refnum<visa-resource-name>)  [unwired: 5 in, 1 out]
                          n215 = Unbundle(w407) -> ("Data"=w401:i32)  [unwired: 2 out]
                          n216 = VISA Flush I/O Buffer(VISA resource name=w408, error in (no error)=w406) -> (error out=w399:errorcluster)  [unwired: 1 in, 1 out]
                          n217 = local write "x [1E-7m]"(w401) -> ()
                        }
                        frame #2 {
                          n218 = local read "z [1E-7m]"() -> (w436:i32)
                          n219 = local read "y [1E-7m]"() -> (w435:i32)
                          n220 = local read "x [1E-7m]"() -> (w434:i32)
                          n221 = Wait (ms)(milliseconds to wait=u32 500 ("millisecond timer value")) -> ()  [unwired: 1 out]
                          n222 = Build Array(w436, w435, w434) -> (w433:i32[])
                          n223 = Less Or Equal?(x=w433, y=2) -> (x <= y?=w432:bool[])
                          n224 = case shown="True" w437 {
                            frame False {
                            }
                            frame True {
                              n225 = call "Display Message to User3"() -> ("error out"=w439:errorcluster)  [unwired: 10 in, 1 out]
                              n226 = local write "error out Stage"(w439) -> ()
                            }
                          }
                          n227 = Or Array Elements(Boolean array=w432) -> (logical OR=w430:bool)
                        }
                      }
                    }
                  }
                }
              }
              event "Open/Close Shutter": Value Change {
                n228 = event-data() -> ()  [unwired: 1 in, 6 out]
                n229 = case shown="False" w443 {
                  tunnel: [0.0 5.0] -> w441
                  frame False {
                  }
                  frame True {
                  }
                }
                n230 = local read "DAQmx Task Shutter"() -> (w442:refnum<k21>)
                n231 = call-poly <vilib>:"DAQmx Write.vi"("task/channels in"=w442, "data"=w441) -> ("error out"=w440:errorcluster)  [unwired: 11 in, 2 out]
              }
              event "Calc Offset": Value Change {
                n232 = event-data() -> ()  [unwired: 1 in, 6 out]
                n233 = flat-sequence {
                  tunnel: w448 -> [w558]
                  tunnel: [w557] -> w447
                  tunnel: w446 -> [w556]
                  frame #0 {
                    n234 = local read "x 3"() -> (w461:i32)
                    n235 = local read "x 1"() -> (w450:i32)
                    n236 = local read "y 2"() -> (w462:i32)
                    n237 = local read "y 3"() -> (w451:i32)
                    n238 = local read "x 2"() -> (w449:i32)
                    n239 = local read "y 1"() -> (w460:i32)
                    n240 = local read "z 2"() -> (w456:i32)
                    n241 = local read "z 3"() -> (w458:i32)
                    n242 = local read "z 1"() -> (w457:i32)
                    n243 = local read "z 1"() -> (w459:i32)
                    n244 = while {
                      tunnel: w462 -> [w484]
                      tunnel: w461 -> [w486]
                      tunnel: w460 -> [w501]
                      tunnel: w450 -> [w487]
                      tunnel: w449 -> [w502]
                      tunnel: w451 -> [w485]
                      tunnel: w459 -> [w503]
                      tunnel: w458 -> [w488]
                      tunnel: w457 -> [w489]
                      tunnel: w456 -> [w490]
                      tunnel: [w470] -> w455
                      tunnel: [w477] -> w454
                      tunnel: [w469] -> w453
                      tunnel: [w480] -> w452
                      tunnel: w451 -> [w475]
                      tunnel: w450 -> [w473]
                      tunnel: w449 -> [w472]
                      i -> [w491]
                      stop <- w465 continue-if-true
                      n245 = case shown="3" w491 {
                        tunnel: w484 -> [w516 w528 w550 _]
                        tunnel: w486 -> [w520 w527 w551 _]
                        tunnel: [w517 w531 w549 w555] -> w500
                        tunnel: [w518 w532 w548 w555] -> w499
                        tunnel: w501 -> [w509 w524 w541 _]
                        tunnel: w487 -> [w519 _ _ _]
                        tunnel: w502 -> [_ _ w552 _]
                        tunnel: w503 -> [w515 _ w544 _]
                        tunnel: w488 -> [w514 w530 w545 _]
                        tunnel: [w513 w533 w547 w555] -> w498
                        tunnel: w490 -> [w512 w529 w553 _]
                        tunnel: [w511 w534 w546 w555] -> w497
                        tunnel: w489 -> [w510 w537 _ _]
                        tunnel: w487 -> [_ w536 _ _]
                        tunnel: w485 -> [_ w535 _ _]
                        tunnel: w475 -> [w508 w526 w543 _]
                        tunnel: [w507 w525 w542 w554] -> w474
                        tunnel: w473 -> [w505 w523 w539 _]
                        tunnel: w472 -> [w504 w522 w538 _]
                        tunnel: [w506 w521 w540 w554] -> w471
                        frame 0, Default {
                          n246 = Subtract(x=w520, y=w519) -> (x-y=w518:i32)
                          n247 = Subtract(x=w516, y=w509) -> (x-y=w517:i32)
                          n248 = Subtract(x=w508, y=w509) -> (x-y=w507:i32)
                          n249 = Subtract(x=w504, y=w505) -> (x-y=w506:i32)
                          n250 = Subtract(x=w512, y=w510) -> (x-y=w511:i32)
                          n251 = Subtract(x=w514, y=w515) -> (x-y=w513:i32)
                        }
                        frame 1 {
                          n252 = Subtract(x=w527, y=w536) -> (x-y=w532:i32)
                          n253 = Subtract(x=w528, y=w535) -> (x-y=w531:i32)
                          n254 = Subtract(x=w526, y=w524) -> (x-y=w525:i32)
                          n255 = Subtract(x=w522, y=w523) -> (x-y=w521:i32)
                          n256 = Subtract(x=w529, y=w530) -> (x-y=w534:i32)
                          n257 = Subtract(x=w530, y=w537) -> (x-y=w533:i32)
                        }
                        frame 2 {
                          n258 = Subtract(x=w551, y=w552) -> (x-y=w548:i32)
                          n259 = Subtract(x=w550, y=w541) -> (x-y=w549:i32)
                          n260 = Subtract(x=w543, y=w541) -> (x-y=w542:i32)
                          n261 = Subtract(x=w538, y=w539) -> (x-y=w540:i32)
                          n262 = Subtract(x=w553, y=w544) -> (x-y=w546:i32)
                          n263 = Subtract(x=w545, y=w553) -> (x-y=w547:i32)
                        }
                        frame 3 {
                          w554 = 1
                          w555 = 0
                          n264 = call "Warning!"() -> ()  [unwired: 10 in, 2 out]
                        }
                      }
                      n265 = Divide(x=w499, y=w474) -> (x/y=w477:dbl)
                      n266 = Divide(x=w500, y=w471) -> (x/y=w470:dbl)
                      n267 = Divide(x=w497, y=w471) -> (x/y=w480:dbl)
                      n268 = Divide(x=w498, y=w474) -> (x/y=w469:dbl)
                      n269 = Absolute Value(x=w477) -> (abs(x)=w476:dbl)
                      n270 = Not A Number/Path/Refnum?(number/path/refnum=w477) -> (NaN/Path/Refnum?=w466:bool)
                      n271 = Absolute Value(x=w470) -> (abs(x)=w478:dbl)
                      n272 = Not A Number/Path/Refnum?(number/path/refnum=w470) -> (NaN/Path/Refnum?=w468:bool)
                      n273 = Absolute Value(x=w480) -> (abs(x)=w479:dbl)
                      n274 = Not A Number/Path/Refnum?(number/path/refnum=w469) -> (NaN/Path/Refnum?=w467:bool)
                      n275 = Absolute Value(x=w469) -> (abs(x)=w481:dbl)
                      n276 = Greater?(x=w476, y="Maximum offset") -> (0:w496:bool)
                      n277 = Greater?(x=w478, y="Maximum offset") -> (0:w495:bool)
                      n278 = Greater?(x=w479, y="Maximum offset") -> (0:w494:bool)
                      n279 = Greater?(x=w481, y="Maximum offset") -> (0:w493:bool)
                      n280 = Build Array(w466, w468, w467) -> (w463:bool[])
                      n281 = Or Array Elements(Boolean array=w463) -> (logical OR=w464:bool)
                      n282 = Build Array(w496, w495, w493, w494) -> (w483:bool[])
                      n283 = Or Array Elements(Boolean array=w483) -> (logical OR=w482:bool)
                      n284 = Or(x=w482, y=w464) -> (x .or. y?=w465:bool)
                    }
                    n285 = local write "Offset x per µm"(w454) -> ()
                    n286 = local write "Offset y per µm"(w455) -> ()
                    n287 = local write "Offset z(y) per µm"(w452) -> ()
                    n288 = local write "Offset z(x) per µm"(w453) -> ()
                  }
                  frame #1 {
                    n289 = flat-sequence {
                      tunnel: [w595] -> _
                      tunnel: [w597] -> w557
                      tunnel: w558 -> [w594]
                      tunnel: w556 -> [w591]
                      frame #0 {
                        n290 = local read "zs"() -> (w564:i32)
                        n291 = local read "xs"() -> (w563:i32)
                        n292 = local write "position reached"(FALSE ("Blinking")) -> ()
                        n293 = And(x=w564, y=w563) -> (x .and. y?=w562:i32)
                        n294 = local read "ys"() -> (w561:i32)
                        n295 = And(x=w562, y=w561) -> (x .and. y?=w560:i32)
                        n296 = Equal To 0?(x=w560) -> (x = 0?=w559:bool)
                        n297 = case shown="True" w559 {
                          frame False {
                          }
                          frame True {
                            n298 = local read "x 1"() -> (w574:i32)
                            n299 = local read "y 1"() -> (w573:i32)
                            n300 = And(x=w574, y=w573) -> (x .and. y?=w572:i32)
                            n301 = local read "z 1"() -> (w571:i32)
                            n302 = And(x=w572, y=w571) -> (x .and. y?=w570:i32)
                            n303 = Not Equal To 0?(x=w570) -> (x != 0?=w569:bool)
                            n304 = case shown="False" w569 {
                              tunnel: [w577 w590] -> w568
                              tunnel: [w575 w589] -> w567
                              tunnel: [w579 w588] -> w566
                              frame False {
                                n305 = local read "error out Stage"() -> (w583:errorcluster)
                                n306 = call "Warning! You may ruin your measurement."("error in (no error)"=w583) -> ("z"=w580:dbl, "y"=w578:dbl, "x"=w576:dbl, "OK"=w581:bool, "error out"=w582:errorcluster)  [unwired: 14 in]
                                n307 = case shown="False" w581 {
                                tunnel: w580 -> [_ w587]
                                tunnel: [w584 w587] -> w579
                                tunnel: w578 -> [_ w585]
                                tunnel: [w584 w586] -> w577
                                tunnel: w576 -> [_ w586]
                                tunnel: [w584 w585] -> w575
                                frame False {
                                w584 = 0
                                }
                                frame True {
                                }
                                }
                                n308 = local write "error out Stage"(w582) -> ()
                              }
                              frame True {
                                n309 = call "Display Message to User2"() -> ()  [unwired: 10 in, 2 out]
                                n310 = local read "z 1"() -> (w588:i32)
                                n311 = local read "y 1"() -> (w589:i32)
                                n312 = local read "x 1"() -> (w590:i32)
                              }
                            }
                            n313 = local write "zs"(w566) -> ()
                            n314 = local write "ys"(w567) -> ()
                            n315 = local write "xs"(w568) -> ()
                          }
                        }
                      }
                      frame #1 {
                        n316 = Wait (ms)(milliseconds to wait=u32 500 ("millisecond timer value")) -> ()  [unwired: 1 out]
                        n317 = local read "zs"() -> (w593:i32)
                        n318 = local read "xs"() -> (w606:i32)
                        n319 = local read "ys"() -> (w617:i32)
                        n320 = Bundle By Name(cluster=w591, "Device Number"=u8 1, "Command"=u8 20, "Data"=w593) -> (w601:T1)
                        n321 = Bundle By Name(cluster=w591, "Device Number"=u8 2, "Command"=u8 20, "Data"=w606) -> (w611:T1)
                        n322 = Bundle By Name(cluster=w591, "Device Number"=u8 3, "Command"=u8 20, "Data"=w617) -> (w614:T1)
                        n323 = call "Request Command.vi"("Request"=w614, "VISA resource name"=w594) -> ("error out"=w616:errorcluster, "VISA resource name out"=w615:refnum<visa-resource-name>)  [unwired: 6 in, 2 out]
                        n324 = VISA Flush I/O Buffer(VISA resource name=w615, error in (no error)=w616) -> (VISA resource name out=w610:refnum<visa-resource-name>, error out=w609:errorcluster)  [unwired: 1 in]
                        n325 = call "Request Command.vi"("error in (no error)"=w609, "Request"=w611, "VISA resource name"=w610) -> ("error out"=w604:errorcluster, "VISA resource name out"=w605:refnum<visa-resource-name>)  [unwired: 5 in, 2 out]
                        n326 = VISA Flush I/O Buffer(VISA resource name=w605, error in (no error)=w604) -> (VISA resource name out=w598:refnum<visa-resource-name>, error out=w596:errorcluster)  [unwired: 1 in]
                        n327 = call "Request Command.vi"("error in (no error)"=w596, "Request"=w601, "VISA resource name"=w598) -> ("error out"=w599:errorcluster, "VISA resource name out"=w600:refnum<visa-resource-name>)  [unwired: 5 in, 2 out]
                        n328 = VISA Flush I/O Buffer(VISA resource name=w600, error in (no error)=w599) -> (VISA resource name out=w595:refnum<visa-resource-name>, error out=w597:errorcluster)  [unwired: 1 in]
                      }
                      frame #2 {
                        n329 = local read "zs"() -> (w618:i32)
                        n330 = local read "ys"() -> (w620:i32)
                        n331 = local read "xs"() -> (w619:i32)
                        n332 = local write "position reached"(TRUE ("Blinking")) -> ()
                        n333 = local write "z [1E-7m]"(w618) -> ()
                        n334 = local write "x [1E-7m]"(w619) -> ()
                        n335 = local write "y [1E-7m]"(w620) -> ()
                      }
                    }
                  }
                }
              }
            }
            n336 = local write "error out shutter"(w141) -> ()
            n337 = local write "error out Stage"(w144) -> ()
            n338 = local write "error out Laserdiode"(w140) -> ()
            n339 = local read "Stop Button"() -> (w147:bool)
          }
          n340 = while {
            tunnel: [w625] -> w137
            tunnel: "Request 11" -> [w624]
            tunnel: w135 -> [w623]
            tunnel: [w622] -> w134
            stop <- "End measurement" stop-if-true
            n341 = Wait (ms)(milliseconds to wait=u32 10000) -> ()  [unwired: 1 out]
            n342 = case shown="True" "Begin measurement" {
              tunnel: [w630 w667] -> w625
              tunnel: w624 -> [_ w665]
              tunnel: w623 -> [w629 w664]
              tunnel: [w629 w663] -> w622
              frame False {
                n343 = while {
                  stop <- w631 stop-if-true
                  n344 = flat-sequence {
                    tunnel: [w635] -> w631
                    frame #0 {
                      n345 = local read "Open/Close Shutter"() -> (w639:bool)
                      n346 = local read "Turn on / off"() -> (w633:bool)
                      n347 = local read "Begin measurement"() -> (w634:bool)
                      n348 = Not(x=w639) -> (.not. x?=w640:bool)
                      n349 = And(x=w633, y=w640) -> (x .and. y?=w641:bool)
                      n350 = local read "stop Shutter"() -> (w638:bool)
                      n351 = And(x=w634, y=w641) -> (x .and. y?=w642:bool)
                      n352 = local read "End measurement"() -> (w637:bool)
                      n353 = Or(x=w642, y=w638) -> (x .or. y?=w636:bool)
                      n354 = Or(x=w637, y=w636) -> (x .or. y?=w635:bool)
                    }
                  }
                  n355 = Wait Until Next ms Multiple(millisecond multiple=u32 500) -> ()  [unwired: 1 out]
                }
                n356 = local read "error out Stage"() -> (w630:errorcluster)
              }
              frame True {
                n357 = local read "zs"() -> (→"z(x) corrected":i32)
                n358 = local read "xs"() -> (→"x corrected":i32)
                n359 = Not A Number/Path/Refnum?(number/path/refnum="File Export Path") -> (NaN/Path/Refnum?=w662:bool)
                n360 = case shown="False" w662 {
                  tunnel: [w670 w678] -> w657
                  tunnel: "File Export Path" -> [_ w678]
                  frame False {
                    n361 = Format Date/Time String(time format string (%c)="%m%d%y_%H%M%S") -> (date/time string=w677:string)  [unwired: 2 in]
                    n362 = Concatenate Strings("DataFile_", w677, ".csv" ("string")) -> (w676:string)
                    n363 = String To Path(string=w676) -> (path=w672:path)
                    n364 = call <vilib>:"Dflt Data Dir.vi"() -> ("App:Default Data Directory"=w671:path)
                    n365 = Build Path(base path=w671, name or relative path=w672) -> (appended path=w670:path)
                  }
                  frame True {
                  }
                }
                n366 = local read "ys"() -> (w653:i32)
                n367 = local read "xs"() -> (w652:i32)
                n368 = Add(x="scan range x [1E-7m]", y=w652) -> (x+y=w649:dbl)
                n369 = Add(x="scan range y [1E-7m]", y=w653) -> (x+y=w646:dbl)
                n370 = Build Array(string[] ["x / µm", "y / µm"] ("1D data")) -> (w660:string[][])
                n371 = In Range and Coerce(upper limit=282879.0, x=w646, lower limit=0.0) -> (coerced(x)=w645:dbl)  [unwired: 1 out]
                n372 = In Range and Coerce(upper limit=282879.0, x=w649, lower limit=0.0) -> (coerced(x)=w644:dbl)  [unwired: 1 out]
                n373 = flat-sequence {
                  tunnel: [w687] -> w669
                  tunnel: [w686] -> w668
                  tunnel: [w685] -> w666
                  tunnel: w665 -> [w684]
                  tunnel: w664 -> [w683]
                  tunnel: w657 -> [w682]
                  tunnel: w645 -> [w681]
                  tunnel: w644 -> [w680]
                  tunnel: w669 -> [w1108]
                  tunnel: w668 -> [w1107]
                  tunnel: [w1106] -> w667
                  tunnel: w666 -> [w1105]
                  tunnel: [w1104] -> w663
                  frame #0 {
                    n374 = local read "WriteMS"() -> (w679:bool)
                    n375 = while {
                      tunnel: [w708] -> w687
                      tunnel: [w706] -> w686
                      tunnel: [w703] -> w685
                      tunnel: w684 -> [w702]
                      tunnel: w683 -> [w701]
                      tunnel: w682 -> [w700]
                      tunnel: w681 -> [w698]
                      tunnel: w680 -> [w697]
                      tunnel: w679 -> [w694]
                      stop <- w709 stop-if-true
                      n376 = flat-sequence {
                        tunnel: w694 -> [w712]
                        tunnel: w697 -> [w713]
                        tunnel: w698 -> [w714]
                        tunnel: w700 -> [w715]
                        tunnel: w701 -> [w716]
                        tunnel: w702 -> [w717]
                        tunnel: [w717] -> w693
                        tunnel: [w716] -> w692
                        tunnel: [w715] -> w691
                        tunnel: [w714] -> w690
                        tunnel: [w713] -> w689
                        tunnel: [w712] -> w688
                        tunnel: [w740] -> w707
                        tunnel: [w739] -> w705
                        tunnel: [w738] -> w704
                        tunnel: [w732] -> w696
                        tunnel: [w731] -> w695
                        tunnel: w693 -> [w737]
                        tunnel: w692 -> [w736]
                        tunnel: w691 -> [w735]
                        tunnel: w690 -> [w734]
                        tunnel: w689 -> [w733]
                        tunnel: w688 -> [_]
                        tunnel: [w1037] -> w708
                        tunnel: w707 -> [w1036]
                        tunnel: [w1035] -> w706
                        tunnel: w705 -> [w1034]
                        tunnel: w704 -> [w1033]
                        tunnel: [w1032] -> w703
                        tunnel: w696 -> [w1031]
                        tunnel: w695 -> [w1030]
                        frame #0 {
                          n377 = case shown="True" w712 {
                            frame False {
                            }
                            frame True {
                              n378 = flat-sequence {
                                tunnel: [w722] -> w719
                                tunnel: [w721] -> w718
                                tunnel: w718 -> [w728]
                                tunnel: w719 -> [w729]
                                frame #0 {
                                n379 = local read "DAQmx Task MS"() -> (w724:refnum<k21>)
                                n380 = local write "WriteMS"(FALSE) -> ()
                                n381 = Wait (ms)(milliseconds to wait=u32 600) -> ()  [unwired: 1 out]
                                n382 = call-poly <vilib>:"DAQmx Write.vi"("task/channels in"=w724, "data"=TRUE) -> ("task out"=w722:refnum<k21>, "error out"=w721:errorcluster)  [unwired: 11 in, 1 out]
                                }
                                frame #1 {
                                n383 = Wait (ms)(milliseconds to wait=u32 100 ("millisecond timer value")) -> ()  [unwired: 1 out]
                                n384 = call-poly <vilib>:"DAQmx Write.vi"("task/channels in"=w729, "data"=FALSE, "error in"=w728) -> ("error out"=w727:errorcluster)  [unwired: 10 in, 2 out]
                                n385 = local write "error out MS"(w727) -> ()
                                }
                              }
                            }
                          }
                        }
                        frame #1 {
                          # "should not change in a measurement"
                          n386 = while {
                            tunnel: "step scanning or continous (scan speed)" -> [w757]
                            tunnel: [w756] -> w740
                            tunnel: [w755] -> w739
                            tunnel: [w751] -> w738
                            tunnel: w737 -> [w750]
                            tunnel: w736 -> [w749]
                            tunnel: w735 -> [w746]
                            tunnel: w734 -> [w742]
                            tunnel: w733 -> [w745]
                            tunnel: [w744] -> w732
                            tunnel: [w743] -> w731
                            stop <- w760 stop-if-true
                            n387 = local read "y [1E-7m]"() -> (w759:i32)
                            n388 = local read "End measurement"() -> (w761:bool)
                            n389 = Equal?(x=w759, y=w742) -> (x = y?=w747:bool)
                            n390 = Or(x=w747, y=w761) -> (x .or. y?=w760:bool)
                            n391 = Not(x=w747) -> (.not. x?=w748:bool)
                            n392 = flat-sequence {
                              tunnel: w747 -> [w775]
                              tunnel: [w775] -> w758
                              tunnel: w757 -> [w774]
                              tunnel: [w773] -> w754
                              tunnel: [w772] -> w753
                              tunnel: [w770] -> w752
                              tunnel: w750 -> [w769]
                              tunnel: w749 -> [w768]
                              tunnel: w748 -> [w767]
                              tunnel: w746 -> [w766]
                              tunnel: w745 -> [w765]
                              tunnel: [w764] -> w744
                              tunnel: [w763] -> w743
                              tunnel: w742 -> [w762]
                              tunnel: w758 -> [w985]
                              tunnel: [w984] -> w756
                              tunnel: [w983] -> w755
                              tunnel: w754 -> [w982]
                              tunnel: w753 -> [w981]
                              tunnel: w752 -> [w980]
                              tunnel: [w979] -> w751
                              frame #0 {
                                n393 = local read "DAQmx Task Shutter"() -> (w771:refnum<k21>)
                                n394 = case shown="True" w774 {
                                tunnel: w769 -> [w786 w882]
                                tunnel: w768 -> [w785 w881]
                                tunnel: [w784 w880] -> w773
                                tunnel: [w783 w877] -> w772
                                tunnel: w771 -> [w782 w879]
                                tunnel: [w781 w878] -> w770
                                tunnel: w767 -> [_ w876]
                                tunnel: w766 -> [w779 w868]
                                tunnel: w765 -> [w778 w875]
                                tunnel: [w777 w875] -> w764
                                tunnel: [w776 w874] -> w763
                                tunnel: w762 -> [w776 w874]
                                frame False {
                                # "1.1% stage error"
                                # "200µm = ca 2000 in steps"
                                # "y+step+offset in y axis (e.g. if the spots are not on a single line)"
                                # "y+step+offset in x-axis is ok though (the offset measured on the axis moving, i.e. offset in x, when moved in y)"
                                n395 = flat-sequence {
                                tunnel: [w811] -> w789
                                tunnel: [w810] -> w788
                                tunnel: w779 -> [w790]
                                tunnel: w782 -> [w808]
                                tunnel: "Shutter time (ms)" -> [w809]
                                tunnel: w789 -> [w816]
                                tunnel: w788 -> [w815]
                                tunnel: "y = step height [1E-7m]" -> [w826]
                                tunnel: w786 -> [w833]
                                tunnel: w785 -> [w835]
                                tunnel: [w825] -> w784
                                tunnel: [w834] -> w783
                                tunnel: [w833] -> w781
                                tunnel: w776 -> [w821]
                                tunnel: w778 -> [w819]
                                tunnel: [w819] -> w777
                                frame #0 {
                                n396 = Wait (ms)(milliseconds to wait=w809) -> ()  [unwired: 1 out]
                                n397 = local write "Open/Close Shutter"(TRUE) -> ()
                                n398 = local read "x corrected"() -> (w807:i32)
                                n399 = local read "y [1E-7m]"() -> (w806:i32)
                                n400 = local read "xs"() -> (w804:i32)
                                n401 = local read "ys"() -> (w805:i32)
                                n402 = Subtract(x=w807, y=w804) -> (x-y=w801:i32)
                                n403 = Subtract(x=w806, y=w805) -> (x-y=w799:i32)
                                n404 = Divide(x=w801, y=10.0) -> (x/y=w800:dbl)
                                n405 = Divide(x=w799, y=10.0) -> (x/y=w798:dbl)
                                n406 = Build Array(w800, w798) -> (w803:T3)
                                n407 = call-poly <vilib>:"Matrix To Array.vi"("Real Matrix"=w803) -> ("Real 2D Array"=w802:dbl[][])
                                n408 = Number To Fractional String(number=w802, precision (6)=i16 1) -> (F-format string=w797:string[][])  [unwired: 2 in]
                                n409 = Reshape Array(w797, 2 ("dimension size")) -> (w796:string[])
                                n410 = call-poly <vilib>:"DAQmx Write.vi"("task/channels in"=w808, "data"=5.0) -> ("task out"=w810:refnum<k21>, "error out"=w811:errorcluster)  [unwired: 11 in, 1 out]
                                n411 = call-poly <vilib>:"Write Delimited Spreadsheet.vi"("file path (dialog if empty)"=w790, "1D data"=w796, "append to file? (new file:F)"=TRUE) -> ()  [unwired: 11 in, 2 out]
                                }
                                frame #1 {
                                n412 = local write "Open/Close Shutter"(FALSE) -> ()
                                n413 = call-poly <vilib>:"DAQmx Write.vi"("task/channels in"=w815, "data"=0.0, "error in"=w816) -> ("error out"=w814:errorcluster)  [unwired: 10 in, 2 out]
                                n414 = local write "error out shutter"(w814) -> ()
                                }
                                frame #2 {
                                # "Offset cannot be saved, as the variable is required for offset calculation. Another indicator is required for that."
                                # "Correct z in a) offset in this step and b) offsets from the next step.\nSee info w/ shift registers.."
                                # "x is corrected by the offset in this step. Correction for every x step already taken is performed in the next step. This can\nbe done properly with shift registers, but I realized too late. See comment above. Correct?"
                                # "y is mainly moving"
                                n415 = Wait (ms)(milliseconds to wait=u32 500) -> ()  [unwired: 1 out]
                                n416 = Multiply(x=w826, y=0.011) -> (x*y=w827:dbl)
                                n417 = Add(x=w826, y=w827) -> (x+y=w828:dbl)
                                n418 = local read "y [1E-7m]"() -> (w832:i32)
                                n419 = Add(x=w828, y=w832) -> (x+y=w831:dbl)
                                n420 = In Range and Coerce(upper limit=w821, x=w831, lower limit=0.0) -> (coerced(x)=w823:dbl)  [unwired: 1 out]
                                n421 = local read "Offset z(x) per µm"() -> (w837:dbl)
                                n422 = local read "Offset x per µm"() -> (w860:dbl)
                                n423 = local write "y [1E-7m]"(w823) -> ()
                                n424 = local read "ys"() -> (w824:i32)
                                n425 = Subtract(x=w823, y=w824) -> (x-y=w830:dbl)
                                n426 = local read "z [1E-7m]"() -> (w845:i32)
                                n427 = Multiply(x=w860, y=w830) -> (x*y=w846:dbl)
                                n428 = Multiply(x=w830, y=w837) -> (x*y=w843:dbl)
                                n429 = Add(x=w843, y=w845) -> (x+y=w844:dbl)
                                n430 = local read "x [1E-7m]"() -> (w838:i32)
                                n431 = In Range and Coerce(upper limit=282879.0, x=w844, lower limit=0.0) -> (coerced(x)=w822:dbl)  [unwired: 1 out]
                                n432 = Add(x=w838, y=w846) -> (x+y=w836:dbl)
                                n433 = local write "z(x) corrected"(w822) -> ()
                                n434 = In Range and Coerce(upper limit=w819, x=w836, lower limit=0.0) -> (coerced(x)=w820:dbl)  [unwired: 1 out]
                                n435 = local write "x corrected"(w820) -> ()
                                n436 = Bundle By Name(cluster=w833, "Device Number"=u8 3, "Command"=u8 20, "Data"=w823) -> (w867:T1)
                                n437 = Bundle By Name(cluster=w833, "Device Number"=u8 1, "Command"=u8 20, "Data"=w822) -> (w854:T1)
                                n438 = call "Request Command.vi"("Request"=w854, "VISA resource name"=w835) -> ("error out"=w852:errorcluster, "VISA resource name out"=w853:refnum<visa-resource-name>)  [unwired: 6 in, 2 out]
                                n439 = Bundle By Name(cluster=w833, "Device Number"=u8 2, "Command"=u8 20, "Data"=w820) -> (w857:T1)
                                n440 = VISA Flush I/O Buffer(VISA resource name=w853, error in (no error)=w852) -> (VISA resource name out=w840:refnum<visa-resource-name>, error out=w842:errorcluster)  [unwired: 1 in]
                                n441 = call "Request Command.vi"("error in (no error)"=w842, "Request"=w857, "VISA resource name"=w840) -> ("error out"=w855:errorcluster, "VISA resource name out"=w856:refnum<visa-resource-name>)  [unwired: 5 in, 2 out]
                                n442 = VISA Flush I/O Buffer(VISA resource name=w856, error in (no error)=w855) -> (VISA resource name out=w839:refnum<visa-resource-name>, error out=w841:errorcluster)  [unwired: 1 in]
                                n443 = call "Request Command.vi"("error in (no error)"=w841, "Request"=w867, "VISA resource name"=w839) -> ("error out"=w866:errorcluster, "VISA resource name out"=w865:refnum<visa-resource-name>)  [unwired: 5 in, 2 out]
                                n444 = VISA Flush I/O Buffer(VISA resource name=w865, error in (no error)=w866) -> (VISA resource name out=w834:refnum<visa-resource-name>, error out=w825:errorcluster)  [unwired: 1 in]
                                }
                                }
                                }
                                frame True {
                                w869 = 282879.0
                                n445 = local read "scan range y [1E-7m]"() -> (w872:dbl)
                                n446 = local read "ys"() -> (w873:i32)
                                n447 = Add(x=w873, y=w872) -> (x+y=w871:dbl)
                                n448 = Less Or Equal?(x=w871, y=w869) -> (x <= y?=w870:bool)
                                n449 = case shown="True" w876 {
                                tunnel: w882 -> [w885 w896]
                                tunnel: w881 -> [w883 w895]
                                tunnel: [w884 w892] -> w880
                                tunnel: [w883 w891] -> w877
                                tunnel: w879 -> [_ w894]
                                tunnel: [w885 w893] -> w878
                                tunnel: w874 -> [_ w890]
                                tunnel: w870 -> [_ w889]
                                tunnel: w869 -> [_ w887]
                                tunnel: w868 -> [_ w886]
                                frame False {
                                n450 = local read "error out Stage"() -> (w884:errorcluster)
                                }
                                frame True {
                                n451 = flat-sequence {
                                tunnel: [w925] -> w906
                                tunnel: [w924] -> w905
                                tunnel: w894 -> [w923]
                                tunnel: w889 -> [w922]
                                tunnel: [w921] -> w888
                                tunnel: w887 -> [w920]
                                tunnel: w886 -> [w907]
                                tunnel: [w945] -> w904
                                tunnel: w896 -> [w945]
                                tunnel: w895 -> [w944]
                                tunnel: [w943] -> w903
                                tunnel: [w942] -> w902
                                tunnel: w906 -> [w941]
                                tunnel: [w941] -> w901
                                tunnel: w905 -> [w940]
                                tunnel: [w940] -> w900
                                tunnel: w888 -> [w932]
                                tunnel: w904 -> [w969]
                                tunnel: w903 -> [w967]
                                tunnel: w902 -> [w966]
                                tunnel: w901 -> [w971]
                                tunnel: w900 -> [w970]
                                tunnel: [w966] -> w899
                                tunnel: [w967] -> w898
                                tunnel: [w969] -> w897
                                tunnel: [w978] -> w893
                                tunnel: w899 -> [w976]
                                tunnel: w898 -> [w977]
                                tunnel: w897 -> [w978]
                                tunnel: [w976] -> w892
                                tunnel: [w977] -> w891
                                tunnel: w890 -> [w975]
                                frame #0 {
                                n452 = case shown="False" w922 {
                                tunnel: [w928 w931] -> w921
                                tunnel: w920 -> [w930 _]
                                frame False {
                                n453 = local read "ys"() -> (w929:i32)
                                n454 = Subtract(x=w930, y=w929) -> (x-y=w928:dbl)
                                }
                                frame True {
                                n455 = local read "scan range y [1E-7m]"() -> (w931:dbl)
                                }
                                }
                                n456 = local write "Open/Close Shutter"(TRUE) -> ()
                                n457 = local read "x corrected"() -> (w919:i32)
                                n458 = local read "xs"() -> (w918:i32)
                                n459 = Subtract(x=w919, y=w918) -> (x-y=w917:i32)
                                n460 = Divide(x=w917, y=10.0) -> (x/y=w915:dbl)
                                n461 = Build Array(w915) -> (w914:T3)
                                n462 = call-poly <vilib>:"Matrix To Array.vi"("Real Matrix"=w914) -> ("Real 2D Array"=w913:dbl[][])
                                n463 = Number To Fractional String(number=w913, precision (6)=1) -> (F-format string=w911:string[][])  [unwired: 2 in]
                                n464 = Reshape Array(w911, 2) -> (w908:string[])
                                n465 = call-poly <vilib>:"DAQmx Write.vi"("task/channels in"=w923, "data"=5.0) -> ("task out"=w924:refnum<k21>, "error out"=w925:errorcluster)  [unwired: 11 in, 1 out]
                                n466 = call-poly <vilib>:"Write Delimited Spreadsheet.vi"("file path (dialog if empty)"=w907, "1D data"=w908, "append to file? (new file:F)"=TRUE) -> ()  [unwired: 11 in, 2 out]
                                }
                                frame #1 {
                                # "The offset correction with constant movement is tricky, as it's based on absolute position."
                                # "y is mainly moving"
                                n467 = Divide(x=w932, y=9.375) -> (x/y=w938:dbl)
                                n468 = local read "Offset z(x) per µm"() -> (w934:dbl)
                                n469 = local read "Offset x per µm"() -> (w935:dbl)
                                n470 = Divide(x=w938, y="Scan speed in µm/s") -> (x/y=w964:dbl)
                                n471 = Multiply(x=w934, y="Scan speed in µm/s") -> (x*y=w937:dbl)
                                n472 = Multiply(x=w935, y="Scan speed in µm/s") -> (x*y=w936:dbl)
                                n473 = Multiply(x=w964, y=1000) -> (x*y=w965:dbl)
                                n474 = Bundle By Name(cluster=w945, "Device Number"=u8 1, "Command"=u8 22, "Data"=w937) -> (w948:T1)
                                n475 = Bundle By Name(cluster=w945, "Device Number"=u8 2, "Command"=u8 22, "Data"=w936) -> (w954:T1)
                                n476 = Bundle By Name(cluster=w945, "Device Number"=u8 3, "Command"=u8 22, "Data"="Scan speed in µm/s") -> (w953:T1)
                                n477 = Wait (ms)(milliseconds to wait=w965) -> ()  [unwired: 1 out]
                                n478 = call "Request Command.vi"("Request"=w948, "VISA resource name"=w944) -> ("error out"=w952:errorcluster, "VISA resource name out"=w951:refnum<visa-resource-name>)  [unwired: 6 in, 2 out]
                                n479 = call "Request Command.vi"("Request"=w954, "VISA resource name"=w944) -> ("error out"=w957:errorcluster, "VISA resource name out"=w958:refnum<visa-resource-name>)  [unwired: 6 in, 2 out]
                                n480 = VISA Flush I/O Buffer(VISA resource name=w951, error in (no error)=w952) -> (error out=w947:errorcluster)  [unwired: 1 in, 1 out]
                                n481 = VISA Flush I/O Buffer(VISA resource name=w958, error in (no error)=w957) -> (VISA resource name out=w943:refnum<visa-resource-name>, error out=w946:errorcluster)  [unwired: 1 in]
                                n482 = local write "error out Stage"(w947) -> ()
                                n483 = local write "error out Stage"(w946) -> ()
                                n484 = call "Request Command.vi"("Request"=w953, "VISA resource name"=w944) -> ("error out"=w962:errorcluster, "VISA resource name out"=w963:refnum<visa-resource-name>)  [unwired: 6 in, 2 out]
                                n485 = VISA Flush I/O Buffer(VISA resource name=w963, error in (no error)=w962) -> (error out=w942:errorcluster)  [unwired: 1 in, 1 out]
                                }
                                frame #2 {
                                n486 = local write "Open/Close Shutter"(FALSE) -> ()
                                n487 = Wait (ms)(milliseconds to wait=u32 500 ("millisecond timer value")) -> ()  [unwired: 1 out]
                                n488 = call-poly <vilib>:"DAQmx Write.vi"("task/channels in"=w970, "data"=0.0, "error in"=w971) -> ("error out"=w974:errorcluster)  [unwired: 10 in, 2 out]
                                n489 = local write "error out shutter"(w974) -> ()
                                }
                                frame #3 {
                                # "The moving axis must be finished by now, but there is no nice way to read out the current position as far as i know. Dirty set I know.Sorry. Maybe shift register\nwould have been nice here.."
                                # "Readout of x and z does not work every time. Plus, all axis change next step anyway.."
                                n490 = local write "y [1E-7m]"(w975) -> ()
                                }
                                }
                                }
                                }
                                }
                                }
                              }
                              frame #1 {
                                n491 = case shown="True" w985 {
                                tunnel: [w987 w995] -> w984
                                tunnel: [w988 w994] -> w983
                                tunnel: w982 -> [w988 w993]
                                tunnel: w981 -> [w987 w992]
                                tunnel: w980 -> [w986 w991]
                                tunnel: [w986 w991] -> w979
                                frame False {
                                }
                                frame True {
                                n492 = flat-sequence {
                                tunnel: w993 -> [w998]
                                tunnel: w992 -> [w997]
                                tunnel: w991 -> [w996]
                                tunnel: [w1000] -> w990
                                tunnel: [w999] -> w989
                                tunnel: [w1018] -> w994
                                tunnel: [w1019] -> w995
                                tunnel: w990 -> [w1019]
                                tunnel: w989 -> [w1018]
                                frame #0 {
                                # "Still needed for constant movement in y. Prob also good for reset as t = 10s"
                                # "Y steps are done, reset to corrected zero. Stage deviation bilateral is higher, therefore movement\nin one axis only. It also beneficial wrt. to thermal effects"
                                n493 = local read "zs"() -> (w1009:i32)
                                n494 = Bundle By Name(cluster=w996, "Device Number"=u8 1, "Command"=u8 20, "Data"=w1009) -> (w1006:T1)
                                n495 = local write "z [1E-7m]"(w1009) -> ()
                                n496 = Wait (ms)(milliseconds to wait=u32 12000) -> ()  [unwired: 1 out]
                                n497 = local read "ys"() -> (w1015:i32)
                                n498 = call "Request Command.vi"("error in (no error)"=w998, "Request"=w1006, "VISA resource name"=w997) -> ("error out"=w1002:errorcluster, "VISA resource name out"=w1005:refnum<visa-resource-name>)  [unwired: 5 in, 2 out]
                                n499 = Bundle By Name(cluster=w996, "Device Number"=3, "Command"=20, "Data"=w1015) -> (w1014:T1)
                                n500 = local write "y [1E-7m]"(w1015) -> ()
                                n501 = VISA Flush I/O Buffer(VISA resource name=w1005, error in (no error)=w1002) -> (VISA resource name out=w1004:refnum<visa-resource-name>, error out=w1003:errorcluster)  [unwired: 1 in]
                                n502 = call "Request Command.vi"("error in (no error)"=w1003, "Request"=w1014, "VISA resource name"=w1004) -> ("error out"=w1012:errorcluster, "VISA resource name out"=w1013:refnum<visa-resource-name>)  [unwired: 5 in, 2 out]
                                n503 = VISA Flush I/O Buffer(VISA resource name=w1013, error in (no error)=w1012) -> (VISA resource name out=w1000:refnum<visa-resource-name>, error out=w999:errorcluster)  [unwired: 1 in]
                                }
                                frame #1 {
                                n504 = flat-sequence {
                                tunnel: [w1023] -> w1017
                                tunnel: [w1022] -> w1016
                                tunnel: w1017 -> [w1029]
                                tunnel: w1016 -> [w1028]
                                frame #0 {
                                # "Short TTL signal begins the measurement. Instant back to zero, so every measurement is individually triggered\n--> one file per shot or line scan"
                                n505 = Wait (ms)(milliseconds to wait=u32 600) -> ()  [unwired: 1 out]
                                n506 = local read "DAQmx Task MS"() -> (w1024:refnum<k21>)
                                n507 = call-poly <vilib>:"DAQmx Write.vi"("task/channels in"=w1024, "data"=TRUE) -> ("task out"=w1022:refnum<k21>, "error out"=w1023:errorcluster)  [unwired: 11 in, 1 out]
                                }
                                frame #1 {
                                n508 = Wait (ms)(milliseconds to wait=u32 100) -> ()  [unwired: 1 out]
                                n509 = call-poly <vilib>:"DAQmx Write.vi"("task/channels in"=w1028, "data"=FALSE, "error in"=w1029) -> ("error out"=w1027:errorcluster)  [unwired: 10 in, 2 out]
                                n510 = local write "error out MS"(w1027) -> ()
                                }
                                }
                                }
                                }
                                }
                                }
                              }
                            }
                          }
                        }
                        frame #2 {
                          n511 = flat-sequence {
                            tunnel: [w1045] -> w1037
                            tunnel: w1036 -> [w1044]
                            tunnel: [w1043] -> w1035
                            tunnel: w1034 -> [w1042]
                            tunnel: w1033 -> [w1041]
                            tunnel: [w1040] -> w1032
                            tunnel: w1031 -> [w1039]
                            tunnel: w1030 -> [w1038]
                            frame #0 {
                              n512 = local read "End measurement"() -> (w1047:bool)
                              n513 = Not(x=w1047) -> (.not. x?=w1046:bool)
                              n514 = case shown="False" w1046 {
                                tunnel: w1044 -> [w1050 w1100]
                                tunnel: [w1050 w1099] -> w1045
                                tunnel: [w1049 w1098] -> w1043
                                tunnel: w1042 -> [w1049 w1097]
                                tunnel: w1041 -> [w1048 w1096]
                                tunnel: [w1048 w1096] -> w1040
                                tunnel: w1039 -> [_ w1052]
                                tunnel: w1038 -> [_ w1051]
                                frame False {
                                }
                                frame True {
                                # "1.2% stage errror"
                                # "Move x, same corrections for the other two axis"
                                # "Add offset along the x-axis (\"offset y\")"
                                n515 = Wait (ms)(milliseconds to wait=1000) -> ()  [unwired: 1 out]
                                n516 = local read "x [1E-7m]"() -> (w1057:i32)
                                n517 = Multiply(x="x = step width [1E-7m]", y=0.012) -> (x*y=w1056:dbl)
                                n518 = Add(x="x = step width [1E-7m]", y=w1056) -> (x+y=w1058:dbl)
                                n519 = Add(x=w1057, y=w1058) -> (x+y=w1059:dbl)
                                n520 = In Range and Coerce(upper limit=w1052, x=w1059, lower limit=0.0) -> (coerced(x)=w1053:dbl)  [unwired: 1 out]
                                n521 = local write "x corrected"(w1053) -> ()
                                n522 = local read "xs"() -> (w1062:i32)
                                n523 = local write "x [1E-7m]"(w1053) -> ()
                                n524 = local read "Offset z(y) per µm"() -> (w1079:dbl)
                                n525 = Subtract(x=w1053, y=w1062) -> (x-y=w1061:dbl)
                                n526 = local read "Offset y per µm"() -> (w1063:dbl)
                                n527 = Bundle By Name(cluster=w1096, "Device Number"=2, "Command"=20, "Data"=w1053) -> (w1093:T1)
                                n528 = Multiply(x=w1063, y=w1061) -> (x*y=w1064:dbl)
                                n529 = Multiply(x=w1061, y=w1079) -> (x*y=w1067:dbl)
                                n530 = local read "ys"() -> (w1066:i32)
                                n531 = local read "zs"() -> (w1069:i32)
                                n532 = Add(x=w1067, y=w1069) -> (x+y=w1068:dbl)
                                n533 = Add(x=w1066, y=w1064) -> (x+y=w1065:dbl)
                                n534 = In Range and Coerce(upper limit=w1051, x=w1065, lower limit=0.0) -> (coerced(x)=w1055:dbl)  [unwired: 1 out]
                                n535 = local write "y [1E-7m]"(w1055) -> ()
                                n536 = In Range and Coerce(upper limit=282879.0, x=w1068, lower limit=0.0) -> (coerced(x)=w1074:dbl)  [unwired: 1 out]
                                n537 = Bundle By Name(cluster=w1096, "Device Number"=3, "Command"=20, "Data"=w1055) -> (w1085:T1)
                                n538 = local write "z [1E-7m]"(w1074) -> ()
                                n539 = Bundle By Name(cluster=w1096, "Device Number"=u8 1, "Command"=u8 20, "Data"=w1074) -> (w1084:T1)
                                n540 = call "Request Command.vi"("error in (no error)"=w1097, "Request"=w1084, "VISA resource name"=w1100) -> ("error out"=w1082:errorcluster, "VISA resource name out"=w1083:refnum<visa-resource-name>)  [unwired: 5 in, 2 out]
                                n541 = VISA Flush I/O Buffer(VISA resource name=w1083, error in (no error)=w1082) -> (VISA resource name out=w1071:refnum<visa-resource-name>, error out=w1072:errorcluster)  [unwired: 1 in]
                                n542 = call "Request Command.vi"("error in (no error)"=w1072, "Request"=w1093, "VISA resource name"=w1071) -> ("error out"=w1095:errorcluster, "VISA resource name out"=w1094:refnum<visa-resource-name>)  [unwired: 5 in, 2 out]
                                n543 = VISA Flush I/O Buffer(VISA resource name=w1094, error in (no error)=w1095) -> (VISA resource name out=w1070:refnum<visa-resource-name>, error out=w1073:errorcluster)  [unwired: 1 in]
                                n544 = call "Request Command.vi"("error in (no error)"=w1073, "Request"=w1085, "VISA resource name"=w1070) -> ("error out"=w1089:errorcluster, "VISA resource name out"=w1088:refnum<visa-resource-name>)  [unwired: 5 in, 2 out]
                                n545 = VISA Flush I/O Buffer(VISA resource name=w1088, error in (no error)=w1089) -> (VISA resource name out=w1099:refnum<visa-resource-name>, error out=w1098:errorcluster)  [unwired: 1 in]
                                }
                              }
                            }
                          }
                        }
                      }
                      n546 = local read "x [1E-7m]"() -> (w711:i32)
                      n547 = local read "End measurement"() -> (w710:bool)
                      n548 = Equal?(x=w711, y=w697) -> (x = y?=w699:bool)
                      n549 = Or(x=w699, y=w710) -> (x .or. y?=w709:bool)
                    }
                  }
                  frame #1 {
                    # "Reset to corr zero"
                    n550 = local read "ys"() -> (w1109:i32)
                    n551 = local read "zs"() -> (w1103:i32)
                    n552 = local read "xs"() -> (w1102:i32)
                    n553 = local write "Begin measurement"(FALSE) -> ()
                    n554 = local write "WriteMS"(TRUE) -> ()
                    n555 = Bundle By Name(cluster=w1105, "Device Number"=3, "Command"=20, "Data"=w1109) -> (w1126:T1)
                    n556 = local write "z [1E-7m]"(w1103) -> ()
                    n557 = local write "z(x) corrected"(w1103) -> ()
                    n558 = local write "x [1E-7m]"(w1102) -> ()
                    n559 = Bundle By Name(cluster=w1105, "Device Number"=u8 1, "Command"=u8 20, "Data"=w1103) -> (w1121:T1)
                    n560 = local write "y [1E-7m]"(w1109) -> ()
                    n561 = call "Request Command.vi"("error in (no error)"=w1107, "Request"=w1121, "VISA resource name"=w1108) -> ("error out"=w1123:errorcluster, "VISA resource name out"=w1122:refnum<visa-resource-name>)  [unwired: 5 in, 2 out]
                    n562 = VISA Flush I/O Buffer(VISA resource name=w1122, error in (no error)=w1123) -> (VISA resource name out=w1113:refnum<visa-resource-name>, error out=w1118:errorcluster)  [unwired: 1 in]
                    n563 = local write "x corrected"(w1102) -> ()
                    n564 = Bundle By Name(cluster=w1105, "Device Number"=u8 2, "Command"=u8 20, "Data"=w1102) -> (w1115:T1)
                    n565 = call "Request Command.vi"("error in (no error)"=w1118, "Request"=w1115, "VISA resource name"=w1113) -> ("error out"=w1117:errorcluster, "VISA resource name out"=w1114:refnum<visa-resource-name>)  [unwired: 5 in, 2 out]
                    n566 = VISA Flush I/O Buffer(VISA resource name=w1114, error in (no error)=w1117) -> (VISA resource name out=w1112:refnum<visa-resource-name>, error out=w1116:errorcluster)  [unwired: 1 in]
                    n567 = call "Request Command.vi"("error in (no error)"=w1116, "Request"=w1126, "VISA resource name"=w1112) -> ("error out"=w1127:errorcluster, "VISA resource name out"=w1128:refnum<visa-resource-name>)  [unwired: 5 in, 2 out]
                    n568 = VISA Flush I/O Buffer(VISA resource name=w1128, error in (no error)=w1127) -> (VISA resource name out=w1104:refnum<visa-resource-name>, error out=w1106:errorcluster)  [unwired: 1 in]
                  }
                }
                n569 = call-poly <vilib>:"Write Delimited Spreadsheet.vi"("file path (dialog if empty)"=w657, "2D data"=w660, "append to file? (new file:F)"=TRUE) -> ()  [unwired: 11 in, 2 out]
              }
            }
          }
        }
        frame #1 {
          # "sets output voltage to zero after execution"
          # "sets output voltage to zero after execution"
          n570 = call "Close.vi"("error in (no error)"=w1147, "VISA resource name"=w1146) -> ("error out"=w1148:errorcluster)  [unwired: 8 in, 1 out]
          n571 = local read "DAQmx Task MS"() -> (w1136:refnum<k21>)
          n572 = local read "DAQmx Task Name Diode"() -> (w1149:refnum<k21>)
          n573 = local read "DAQmx Task Shutter"() -> (w1152:refnum<k21>)
          n574 = call-poly <vilib>:"DAQmx Write.vi"("task/channels in"=w1136, "data"=FALSE) -> ("task out"=w1131:refnum<k21>, "error out"=w1132:errorcluster)  [unwired: 11 in, 1 out]
          n575 = call-poly <vilib>:"DAQmx Write.vi"("task/channels in"=w1149, "data"=0.0) -> ("task out"=w1144:refnum<k21>, "error out"=w1142:errorcluster)  [unwired: 11 in, 1 out]
          n576 = call <vilib>:"DAQmx Stop Task.vi"("task/channels in"=w1131, "error in"=w1132) -> ("task out"=w1134:refnum<k21>, "error out"=w1133:errorcluster)  [unwired: 12 in]
          n577 = call <vilib>:"DAQmx Clear Task.vi"("task in"=w1134, "error in"=w1133) -> ("error out"=w1130:errorcluster)  [unwired: 13 in]
          n578 = call <vilib>:"DAQmx Stop Task.vi"("task/channels in"=w1144, "error in"=w1142) -> ("task out"=w1143:refnum<k21>, "error out"=w1141:errorcluster)  [unwired: 12 in]
          n579 = call-poly <vilib>:"DAQmx Write.vi"("task/channels in"=w1152, "data"=0.0) -> ("task out"=w1140:refnum<k21>, "error out"=w1138:errorcluster)  [unwired: 11 in, 1 out]
          n580 = local write "error out Stage"(w1148) -> ()
          n581 = call <vilib>:"DAQmx Clear Task.vi"("task in"=w1143, "error in"=w1141) -> ("error out"=w1145:errorcluster)  [unwired: 13 in]
          n582 = local write "error out MS"(w1130) -> ()
          n583 = local write "error out Laserdiode"(w1145) -> ()
          n584 = call <vilib>:"DAQmx Stop Task.vi"("task/channels in"=w1140, "error in"=w1138) -> ("task out"=w1139:refnum<k21>, "error out"=w1137:errorcluster)  [unwired: 12 in]
          n585 = call <vilib>:"DAQmx Clear Task.vi"("task in"=w1139, "error in"=w1137) -> ("error out"=w1151:errorcluster)  [unwired: 13 in]
          n586 = local write "error out shutter"(w1151) -> ()
        }
      }
    }
  }
